vi "OPC UA Client.vi"(11 "?":T9={"VI refs"=[], "Queues"=[], "[Thumbnails]"=[], "Drag Object Idx"=0, "[Objects]"=[], "Active Object"=0, "Drop Offset"={"Left"=0, "Top"=0}, "Process Name"="", "Main Config"={"Notebook"="", "OPC Module Configs"=[], "Feed Module Configs"=[], "Log File Path"=path "", "TT Module Configs"=[], "DAQ Config"={"Tasks"=[]}, "PT Module Configs"=[], "Scale Module Configs"=[], "Pump Module Configs"=[], "U3 Module Configs"=[{"GUID"="", "Drop Coords"={"Horizontal"=0, "Vertical"=0}, "AI Channel Number"=enum."Default", "Process Name"="", "User name"="", "Queue Name"="", "Input Channel Numeric Alarm Settings"=[]}], "Decoration Module Configs"=[], "Flow Module Configs"=[], "TCU Module Configs"=[], "Steps"=[], "Abort"=FALSE, "DO Module Configs"=[], "PR Module Configs"=[], "SC Module Configs"=[], "AM Module Configs"=[], "Cycle Period"=0.0}, "Campaign Filepath"=path "", "Config Changed?"=FALSE} {"Main Config"."PR Module Configs"."Settings"."PID 2 Parameters"."output range"."output low" format="%.2f"; "Main Config"."PR Module Configs"."Settings"."PID 2 Parameters"."output range"."output high" min=0.0 max=100.0 format="%.2f"; "Main Config"."PR Module Configs"."Settings"."PID 2 Parameters"."PID gains"."derivative time (Td, min)" format="%.3f"; "Main Config"."PR Module Configs"."Settings"."PID 2 Parameters"."PID gains"."integral time (Ti, min)" format="%.3f"; "Main Config"."PR Module Configs"."Settings"."PID 2 Parameters"."PID gains"."proportional gain (Kc)" format="%.3f"; "Main Config"."Steps"."Control" items=["Pump %", "Setpoint"]; "Main Config"."TCU Module Configs"."Settings"."Huber Unistat 410 Settings"."Address" min=0 max=99 format="%02.0f"; "Main Config"."TCU Module Configs"."Settings"."Julabo FP-50 Settings"."Pump Power" min=0 max=8 step=1; "Main Config"."TCU Module Configs"."Settings"."Lauda Settings"."Pump Power" min=0 max=8 step=1; "Main Config"."Flow Module Configs"."Settings"."Bronkhorst M14 Settings"."Smoothing Steps" min=1 step=1; "Main Config"."Flow Module Configs"."Settings"."Bronkhorst M13 Settings"."Smoothing Steps" min=1 step=1; "Main Config"."Pump Module Configs"."Settings"."Ismatech 3 Channel Settings"."Channel Number" min=0 max=3; "Main Config"."Pump Module Configs"."Settings"."Ismatech 3 Channel Settings"."Pump Number" min=1; "Main Config"."Pump Module Configs"."Settings"."ASIA Pump C"."channel" min=0 max=1 step=1; "Main Config"."Pump Module Configs"."Settings"."Masterflex"."Pump Number" min=1.0 max=20.0 step=1.0; "Main Config"."Pump Module Configs"."Settings"."Ismatech"."Pump Number" min=1.0 max=20.0 step=1.0; "Main Config"."Feed Module Configs"."Settings"."Bronkhorst M14 Settings"."Smoothing Steps" min=1 step=1; "Main Config"."Feed Module Configs"."Settings"."Ismatech 3 Channel Settings"."Channel Number" min=0 max=3; "Main Config"."Feed Module Configs"."Settings"."Ismatech 3 Channel Settings"."Pump Number" min=1; "Main Config"."Feed Module Configs"."Settings"."output range"."output low" min=0.0 max=100.0 format="%.2f"; "Main Config"."Feed Module Configs"."Settings"."output range"."output high" format="%.2f"; "Main Config"."Feed Module Configs"."Settings"."PID 2 Parameters"."PID gains"."derivative time (Td, min)" format="%.3f"; "Main Config"."Feed Module Configs"."Settings"."PID 2 Parameters"."PID gains"."integral time (Ti, min)" format="%.3f"; "Main Config"."Feed Module Configs"."Settings"."PID 2 Parameters"."PID gains"."proportional gain (Kc)" format="%.3f"; "Main Config"."Feed Module Configs"."Settings"."Bronkhorst M13 Flow Meter"."Smoothing Steps" min=1 step=1; "Main Config"."Feed Module Configs"."Settings"."ASIA Pump C"."channel" min=0 max=1 step=1; "Main Config"."Feed Module Configs"."Settings"."Ismatech"."Pump Number" min=1.0 max=20.0 step=1.0; "Main Config"."Feed Module Configs"."Settings"."Masterflex"."Pump Number" min=1.0 max=20.0 step=1.0}) -> ()   [LabVIEW 2018, in "OPC UA Total Client.lvlib"]
uses:
  OPC UA Total Client.lvlib
  <vilib>/OPCUA/controls/NodeId.ctl
  <vilib>/OPCUA/controls/OPC UA Variable Node Refnum.ctl
  <vilib>/OPCUA/controls/OPC UA Server Refnum.ctl
  Drag and Drop/State Cluster.ctl
  support/Message Queue/Message Cluster.ctl
  Drag and Drop/Thumbnail Cluster.ctl
  Drag and Drop/Object Cluster.ctl
  <vilib>/Utility/miscctls.llb/LVRectTypeDef.ctl
  Drag and Drop/Object Type Enum.ctl
  <vilib>/Utility/miscctls.llb/LVPositionTypeDef.ctl
  Config Module/Controls/Main Config Cluster.ctl
  OPC Module Config.ctl
  Scale Module Folder/Measure Instrument/State Enum.ctl
  <vilib>/Utility/miscctls.llb/LVPoint32TypeDef.ctl
  OPC Settings.ctl
  Variable Data Cluster.ctl
  <vilib>/OPCUA/controls/OPC UA StatusCode.ctl
  <vilib>/OPCUA/controls/Subscription ID.ctl
  <vilib>/OPCUA/controls/OPC UA Client Refnum.ctl
  <vilib>/OPCUA/controls/Subscription Data Change.ctl
  <vilib>/OPCUA/controls/Data Type.ctl
  OPC Tag Data.ctl
  Feed Module/Controls/Feed Module Config Cluster.ctl
  Feed Module/Controls/Feed Module Settings Cluster.ctl
  Ismatec ISM 831C/Controls/Ismatech ISM831C Settings Cluster.ctl
  Masterflex 7550-30/Controls/Settings Cluster.ctl
  Mettler Toledo/Controls/Settings Cluster.ctl
  Bronkhorst M13 Flow Meter/Settings Cluster.ctl
  Measure Instrument/PID 2 Parameters Cluster.ctl
  Measure Instrument/PID Input Enum.ctl
  Measure Instrument/PID 2 Output Enum.ctl
  Tacmina QI/Tacmina QI DAQ Setting.ctl
  KNF Pump/Settings Cluster plus SIMDOS.ctl
  ASIA Pump/Pump Settings.ctl
  VICI M50 Party Mode/Settings Cluster.ctl
  FLOM Pump/Settings Cluster.ctl
  SSI PR Class/SSI PR or LD Settings Cluster.ctl
  Masterflex 75211/Masterflex 75211 DAQ Setting.ctl
  SSI PR Class/SSI P40 Settings Cluster.ctl
  Ismatec 78001/Ismatec 4083.ctl
  Bronkhorst M14 Flow Meter/Settings Cluster.ctl
  TT Module/Controls/TT Module Config Cluster.ctl
  Tag VIs/Numeric Alarm Settings Cluster.ctl
  Acquisition/Hardware Configuration.ctl
  Acquisition/Task Cluster.ctl
  PT Module/Controls/PT Module Config Cluster.ctl
  Scale Module Folder/Feed Module/Controls/Scale Module Config Cluster.ctl
  Scale Module Folder/Feed Module/Controls/Scale Module Settings Cluster.ctl
  Pump Module Folder/Pump Module Config Cluster.ctl
  Pump Module Folder/Pump Module Settings Cluster.ctl
  LabJack Module/Controls/U3 Module Config Cluster.ctl
  Decoration Module/Decoration Module Config Cluster.ctl
  Flow Module Folder/Feed Module/Controls/Flow Module Config Cluster.ctl
  Flow Module Folder/Feed Module/Controls/Flow Module Settings Cluster.ctl
  TCU Module/TCU Module Folder/TCU Module Config Cluster.ctl
  TCU Module/TCU Module Folder/TCU Module Settings Cluster.ctl
  TCU Module/TCU Module Folder/Measure Instrument/Output Devices.ctl
  Huber TCU/Huber Settings.ctl
  Lauda Integral XT-150 TCU/Lauda Settings.ctl
  Julabo Type 1 TCU/Julabo Type 1 TCU Folder/Julabo FP-50 Settings.ctl
  Huber Unistat 410 TCU/Huber Unistat 410 RS485 Settings.ctl
  D-O Module Folder/Not Sure Where this is Used.ctl
  Sequencing/Squence Control.ctl
  D-O Module Folder/D-O Module Config Cluster.ctl
  D-O Module Folder/Valve Clusters.ctl
  D-O Module Folder/D-O Module Settings Cluster.ctl
  D-O Module Folder/D-O Device Settings Cluster.ctl
  VICI Electronic Actuator/VICI Electronic Actuator Settings.ctl
  Pressure Regulator Control Module/Pressure Regulator/Controls/4-20mA Module Config Cluster.ctl
  Pressure Regulator Control Module/Pressure Regulator/Controls/4-20mA Module Settings Cluster.ctl
  Pressure Transmitter/Pressure Transmitter Device Settings.ctl
  Pressure Reg Module/Pressure Regulator Device Settings.ctl
  Sonicator Module Folder/Feed Module/Controls/Sonicator Module Config Cluster.ctl
  Sonicator Module Folder/Feed Module/Controls/Sonicator Module Settings Cluster.ctl
  Sonic Systems P100/Sonic Systems P100 Settings.ctl
  Agitator Module Folder/Feed Module/Controls/Agitator Module Config Cluster.ctl
  Agitator Module Folder/Feed Module/Controls/Agitator Module Settings Cluster.ctl
  <vilib>/OPCUA/controls/Supported Security Policies.ctl
  Main/Main Queue Cluster.ctl
  <vilib>/OPCUA/controls/Read Variant Result.ctl
  <vilib>/OPCUA/controls/Node Class.ctl
  <vilib>/OPCUA/controls/NodeIds.ctl
  <vilib>/OPCUA/client/Multiple Read Variant.vi
  <vilib>/OPCUA/NI OPC UA Server.lvlib
  <vilib>/regexp/Match Regular Expression.xnode
  OPC UA.lvlib
  Tag VIs/Tag FGV Operation Enum.ctl
  Shared Variables/Dynamic Shared Variables.lvlib
  support/Message Queue/Message Queue.lvlib
  <vilib>/OPCUA/NI OPC UA Client.lvlib
  <vilib>/OPCUA/controls/Write Status.ctl
  <vilib>/OPCUA/controls/Write Variant Request.ctl
  <vilib>/OPCUA/server/Write Double.vi
  <vilib>/OPCUA/client/Multiple Write Variant.vi
  support/Message Queue/Enqueue Message (Single).vi
  <vilib>/OPCUA/client/Multiple Write Int32.vi
  TT Module/TT Module.lvlib
  Masterflex 75211/Masterflex 75211.lvlib
  Masterflex 7550-30/Masterflex 7550-30.lvlib
  Ismatec ISM 831C/Ismatec ISM 831C.lvlib
  Tacmina QI/Tacmina QI.lvlib
  KNF Pump/KNF SIMDOS.lvlib
  VICI M50 Party Mode/VICI M6 M50 Party Mode.lvlib
  FLOM Pump/FLOM Pump.lvlib
  ASIA Pump.lvlib
  Mettler Toledo/Mettler Toledo.lvlib
  Bronkhorst M13 Flow Meter/Bronkhorst M13 Flow Meter.lvlib
  SSI PR Class/SSI PR or LD Pump.lvlib
  SSI PR Class/SSI P40 Pump.lvlib
  Feed Module/Feed Module.lvlib
  DAQ/DAQ.lvlib
  PT Module/PT Module.lvlib
  Scale Module Folder/Scale Module.lvlib
  Pump Module Folder/Pump Module.lvlib
  LabJack Module/U3 Module.lvlib
  Flow Module Folder/Flow Module.lvlib
  Huber TCU/Huber Ministat 230 TCU.lvlib
  Lauda Integral XT-150 TCU/Lauda TCU.lvlib
  Julabo Type 1 TCU/Julabo Type 1 TCU Folder/Julabo Type FP-50 TCU.lvlib
  Huber Unistat 410 TCU/Huber Unistat 410 TCU.lvlib
  TCU Module/TCU Module Folder/TCU Module.lvlib
  Sequencing/Sequencing Library.lvlib
  D-O Module Folder/D-O Module.lvlib
  D-O Module Folder/DIO Valve/VICI Electronic Actuator.lvlib
  Pressure Transmitter/Pressure Transmitter Library.lvlib
  Pressure Reg Module/Pressure Regulator Library.lvlib
  Pressure Regulator Control Module/Pressure Regulator/4-20mA Module.lvlib
  Scale Module Folder/Measure Instrument/Scale Module Engine.lvlib
  Config Module/Config Module.lvlib
  Drag and Drop/Drag and Drop.lvlib
  Ismatec 78001/Ismatec 4308.lvlib
  Bronkhorst M14 Flow Meter/Bronkhorst M14 Flow Meter.lvlib
  Sonicator Module Folder/Sonicator Module.lvlib
  Sonic Systems P100/Sonic Systems P100.lvlib
  Agitator Module Folder/Agitator Module.lvlib
panel:
  out "results 2":T1[](array[typedef]) {"status" items=["Good"=0, "Good_SubscriptionTransferred"=2949120, "Good_CompletesAsynchronously"=3014656, "Good_Overload"=3080192, "Good_Clamped"=3145728, "Good_LocalOverride"=9830400, "Good_EntryInserted"=10616832, "Good_EntryReplaced"=10682368, "Good_NoData"=10813440, "Good_MoreData"=10878976, "Good_CommunicationEvent"=10944512, "Good_ShutdownEvent"=11010048, "Good_CallAgain"=11075584, "Good_NonCriticalTimeout"=11141120, "Good_ResultsMayBeIncomplete"=12189696, "Good_DataIgnored"=14221312, "Uncertain"=1073741824, "Uncertain_ReferenceOutOfServer"=1080819712, "Uncertain_NoCommunicationLastUsableValue"=1083113472, "Uncertain_LastUsableValue"=1083179008, "Uncertain_SubstituteValue"=1083244544, "Uncertain_InitialValue"=1083310080, "Uncertain_SensorNotAccurate"=1083375616, "Uncertain_EngineeringUnitsExceeded"=1083441152, "Uncertain_SubNormal"=1083506688, "Uncertain_DataSubNormal"=1084489728, "Uncertain_ReferenceNotDeleted"=1086062592, "Uncertain_NotAllNodesAvailable"=1086324736, "Bad"=2147483648, "Bad_UnexpectedError"=2147549184, "Bad_InternalError"=2147614720, "Bad_OutOfMemory"=2147680256, "Bad_ResourceUnavailable"=2147745792, "Bad_CommunicationError"=2147811328, "Bad_EncodingError"=2147876864, "Bad_DecodingError"=2147942400, "Bad_EncodingLimitsExceeded"=2148007936, "Bad_UnknownResponse"=2148073472, "Bad_Timeout"=2148139008, "Bad_ServiceUnsupported"=2148204544, "Bad_Shutdown"=2148270080, "Bad_ServerNotConnected"=2148335616, "Bad_ServerHalted"=2148401152, "Bad_NothingToDo"=2148466688, "Bad_TooManyOperations"=2148532224, "Bad_DataTypeIdUnknown"=2148597760, "Bad_CertificateInvalid"=2148663296, "Bad_SecurityChecksFailed"=2148728832, "Bad_CertificateTimeInvalid"=2148794368, "Bad_CertificateIssuerTimeInvalid"=2148859904, "Bad_CertificateHostNameInvalid"=2148925440, "Bad_CertificateUriInvalid"=2148990976, "Bad_CertificateUseNotAllowed"=2149056512, "Bad_CertificateIssuerUseNotAllowed"=2149122048, "Bad_CertificateUntrusted"=2149187584, "Bad_CertificateRevocationUnknown"=2149253120, "Bad_CertificateIssuerRevocationUnknown"=2149318656, "Bad_CertificateRevoked"=2149384192, "Bad_CertificateIssuerRevoked"=2149449728, "Bad_UserAccessDenied"=2149515264, "Bad_IdentityTokenInvalid"=2149580800, "Bad_IdentityTokenRejected"=2149646336, "Bad_SecureChannelIdInvalid"=2149711872, "Bad_InvalidTimestamp"=2149777408, "Bad_NonceInvalid"=2149842944, "Bad_SessionIdInvalid"=2149908480, "Bad_SessionClosed"=2149974016, "Bad_SessionNotActivated"=2150039552, "Bad_SubscriptionIdInvalid"=2150105088, "Bad_RequestHeaderInvalid"=2150236160, "Bad_TimestampsToReturnInvalid"=2150301696, "Bad_RequestCancelledByClient"=2150367232, "Bad_NoCommunication"=2150694912, "Bad_WaitingForInitialData"=2150760448, "Bad_NodeIdInvalid"=2150825984, "Bad_NodeIdUnknown"=2150891520, "Bad_AttributeIdInvalid"=2150957056, "Bad_IndexRangeInvalid"=2151022592, "Bad_IndexRangeNoData"=2151088128, "Bad_DataEncodingInvalid"=2151153664, "Bad_DataEncodingUnsupported"=2151219200, "Bad_NotReadable"=2151284736, "Bad_NotWritable"=2151350272, "Bad_OutOfRange"=2151415808, "Bad_NotSupported"=2151481344, "Bad_NotFound"=2151546880, "Bad_ObjectDeleted"=2151612416, "Bad_NotImplemented"=2151677952, "Bad_MonitoringModeInvalid"=2151743488, "Bad_MonitoredItemIdInvalid"=2151809024, "Bad_MonitoredItemFilterInvalid"=2151874560, "Bad_MonitoredItemFilterUnsupported"=2151940096, "Bad_FilterNotAllowed"=2152005632, "Bad_StructureMissing"=2152071168, "Bad_EventFilterInvalid"=2152136704, "Bad_ContentFilterInvalid"=2152202240, "Bad_FilterOperandInvalid"=2152267776, "Bad_ContinuationPointInvalid"=2152333312, "Bad_NoContinuationPoints"=2152398848, "Bad_ReferenceTypeIdInvalid"=2152464384, "Bad_BrowseDirectionInvalid"=2152529920, "Bad_NodeNotInView"=2152595456, "Bad_ServerUriInvalid"=2152660992, "Bad_ServerNameMissing"=2152726528, "Bad_DiscoveryUrlMissing"=2152792064, "Bad_SempahoreFileMissing"=2152857600, "Bad_RequestTypeInvalid"=2152923136, "Bad_SecurityModeRejected"=2152988672, "Bad_SecurityPolicyRejected"=2153054208, "Bad_TooManySessions"=2153119744, "Bad_UserSignatureInvalid"=2153185280, "Bad_ApplicationSignatureInvalid"=2153250816, "Bad_NoValidCertificates"=2153316352, "Bad_RequestCancelledByRequest"=2153381888, "Bad_ParentNodeIdInvalid"=2153447424, "Bad_ReferenceNotAllowed"=2153512960, "Bad_NodeIdRejected"=2153578496, "Bad_NodeIdExists"=2153644032, "Bad_NodeClassInvalid"=2153709568, "Bad_BrowseNameInvalid"=2153775104, "Bad_BrowseNameDuplicated"=2153840640, "Bad_NodeAttributesInvalid"=2153906176, "Bad_TypeDefinitionInvalid"=2153971712, "Bad_SourceNodeIdInvalid"=2154037248, "Bad_TargetNodeIdInvalid"=2154102784, "Bad_DuplicateReferenceNotAllowed"=2154168320, "Bad_InvalidSelfReference"=2154233856, "Bad_ReferenceLocalOnly"=2154299392, "Bad_NoDeleteRights"=2154364928, "Bad_ServerIndexInvalid"=2154430464, "Bad_ViewIdUnknown"=2154496000, "Bad_TooManyMatches"=2154627072, "Bad_QueryTooComplex"=2154692608, "Bad_NoMatch"=2154758144, "Bad_MaxAgeInvalid"=2154823680, "Bad_HistoryOperationInvalid"=2154889216, "Bad_HistoryOperationUnsupported"=2154954752, "Bad_WriteNotSupported"=2155020288, "Bad_TypeMismatch"=2155085824, "Bad_MethodInvalid"=2155151360, "Bad_ArgumentsMissing"=2155216896, "Bad_TooManySubscriptions"=2155282432, "Bad_TooManyPublishRequests"=2155347968, "Bad_NoSubscription"=2155413504, "Bad_SequenceNumberUnknown"=2155479040, "Bad_MessageNotAvailable"=2155544576, "Bad_InsufficientClientProfile"=2155610112, "Bad_TcpServerTooBusy"=2155675648, "Bad_TcpMessageTypeInvalid"=2155741184, "Bad_TcpSecureChannelUnknown"=2155806720, "Bad_TcpMessageTooLarge"=2155872256, "Bad_TcpNotEnoughResources"=2155937792, "Bad_TcpInternalError"=2156003328, "Bad_TcpEndpointUrlInvalid"=2156068864, "Bad_RequestInterrupted"=2156134400, "Bad_RequestTimeout"=2156199936, "Bad_SecureChannelClosed"=2156265472, "Bad_SecureChannelTokenUnknown"=2156331008, "Bad_SequenceNumberInvalid"=2156396544, "Bad_ConfigurationError"=2156462080, "Bad_NotConnected"=2156527616, "Bad_DeviceFailure"=2156593152, "Bad_SensorFailure"=2156658688, "Bad_OutOfService"=2156724224, "Bad_DeadbandFilterInvalid"=2156789760, "Bad_RefreshInProgress"=2157379584, "Bad_ConditionAlreadyDisabled"=2157445120, "Bad_ConditionDisabled"=2157510656, "Bad_EventIdUnknown"=2157576192, "Bad_NoData"=2157641728, "Bad_DataLost"=2157772800, "Bad_DataUnavailable"=2157838336, "Bad_EntryExists"=2157903872, "Bad_NoEntryExists"=2157969408, "Bad_TimestampNotSupported"=2158034944, "Bad_InvalidArgument"=2158690304, "Bad_ConnectionRejected"=2158755840, "Bad_Disconnect"=2158821376, "Bad_ConnectionClosed"=2158886912, "Bad_InvalidState"=2158952448, "Bad_EndOfStream"=2159017984, "Bad_NoDataAvailable"=2159083520, "Bad_WaitingForResponse"=2159149056, "Bad_OperationAbandoned"=2159214592, "Bad_ExpectedStreamToBlock"=2159280128, "Bad_WouldBlock"=2159345664, "Bad_SyntaxError"=2159411200, "Bad_MaxConnectionsReached"=2159476736, "Bad_RequestTooLarge"=2159542272, "Bad_ResponseTooLarge"=2159607808, "Bad_EventNotAcknowledgeable"=2159738880, "Bad_InvalidTimestampArgument"=2159869952, "Bad_ProtocolVersionUnsupported"=2159935488, "Bad_StateNotActive"=2160001024, "Bad_FilterOperatorInvalid"=2160132096, "Bad_FilterOperatorUnsupported"=2160197632, "Bad_FilterOperandCountMismatch"=2160263168, "Bad_FilterElementInvalid"=2160328704, "Bad_FilterLiteralInvalid"=2160394240, "Bad_IdentityChangeNotSupported"=2160459776, "Bad_NotTypeDefinition"=2160590848, "Bad_ViewTimestampInvalid"=2160656384, "Bad_ViewParameterMismatch"=2160721920, "Bad_ViewVersionInvalid"=2160787456, "Bad_ConditionAlreadyEnabled"=2160852992, "Bad_DialogNotActive"=2160918528, "Bad_DialogResponseInvalid"=2160984064, "Bad_ConditionBranchAlreadyAcked"=2161049600, "Bad_ConditionBranchAlreadyConfirmed"=2161115136, "Bad_ConditionAlreadyShelved"=2161180672, "Bad_ConditionNotShelved"=2161246208, "Bad_ShelvingTimeOutOfRange"=2161311744, "Bad_AggregateListMismatch"=2161377280, "Bad_AggregateNotSupported"=2161442816, "Bad_AggregateInvalidInputs"=2161508352, "Bad_BoundNotFound"=2161573888, "Bad_BoundNotSupported"=2161639424, "Bad_AggregateConfigurationRejected"=2161770496, "Bad_TooManyMonitoredItems"=2161836032]}
  out "browse result":T5(array[cluster]) {"node class" items=["Unspecified"=0, "Object"=1, "Variable"=2, "Method"=4, "Object Type"=8, "Variable Type"=16, "Reference Type"=32, "Data Type"=64, "View"=128]}
  out "results":T1[](array[typedef]) {"status" items=["Good"=0, "Good_SubscriptionTransferred"=2949120, "Good_CompletesAsynchronously"=3014656, "Good_Overload"=3080192, "Good_Clamped"=3145728, "Good_LocalOverride"=9830400, "Good_EntryInserted"=10616832, "Good_EntryReplaced"=10682368, "Good_NoData"=10813440, "Good_MoreData"=10878976, "Good_CommunicationEvent"=10944512, "Good_ShutdownEvent"=11010048, "Good_CallAgain"=11075584, "Good_NonCriticalTimeout"=11141120, "Good_ResultsMayBeIncomplete"=12189696, "Good_DataIgnored"=14221312, "Uncertain"=1073741824, "Uncertain_ReferenceOutOfServer"=1080819712, "Uncertain_NoCommunicationLastUsableValue"=1083113472, "Uncertain_LastUsableValue"=1083179008, "Uncertain_SubstituteValue"=1083244544, "Uncertain_InitialValue"=1083310080, "Uncertain_SensorNotAccurate"=1083375616, "Uncertain_EngineeringUnitsExceeded"=1083441152, "Uncertain_SubNormal"=1083506688, "Uncertain_DataSubNormal"=1084489728, "Uncertain_ReferenceNotDeleted"=1086062592, "Uncertain_NotAllNodesAvailable"=1086324736, "Bad"=2147483648, "Bad_UnexpectedError"=2147549184, "Bad_InternalError"=2147614720, "Bad_OutOfMemory"=2147680256, "Bad_ResourceUnavailable"=2147745792, "Bad_CommunicationError"=2147811328, "Bad_EncodingError"=2147876864, "Bad_DecodingError"=2147942400, "Bad_EncodingLimitsExceeded"=2148007936, "Bad_UnknownResponse"=2148073472, "Bad_Timeout"=2148139008, "Bad_ServiceUnsupported"=2148204544, "Bad_Shutdown"=2148270080, "Bad_ServerNotConnected"=2148335616, "Bad_ServerHalted"=2148401152, "Bad_NothingToDo"=2148466688, "Bad_TooManyOperations"=2148532224, "Bad_DataTypeIdUnknown"=2148597760, "Bad_CertificateInvalid"=2148663296, "Bad_SecurityChecksFailed"=2148728832, "Bad_CertificateTimeInvalid"=2148794368, "Bad_CertificateIssuerTimeInvalid"=2148859904, "Bad_CertificateHostNameInvalid"=2148925440, "Bad_CertificateUriInvalid"=2148990976, "Bad_CertificateUseNotAllowed"=2149056512, "Bad_CertificateIssuerUseNotAllowed"=2149122048, "Bad_CertificateUntrusted"=2149187584, "Bad_CertificateRevocationUnknown"=2149253120, "Bad_CertificateIssuerRevocationUnknown"=2149318656, "Bad_CertificateRevoked"=2149384192, "Bad_CertificateIssuerRevoked"=2149449728, "Bad_UserAccessDenied"=2149515264, "Bad_IdentityTokenInvalid"=2149580800, "Bad_IdentityTokenRejected"=2149646336, "Bad_SecureChannelIdInvalid"=2149711872, "Bad_InvalidTimestamp"=2149777408, "Bad_NonceInvalid"=2149842944, "Bad_SessionIdInvalid"=2149908480, "Bad_SessionClosed"=2149974016, "Bad_SessionNotActivated"=2150039552, "Bad_SubscriptionIdInvalid"=2150105088, "Bad_RequestHeaderInvalid"=2150236160, "Bad_TimestampsToReturnInvalid"=2150301696, "Bad_RequestCancelledByClient"=2150367232, "Bad_NoCommunication"=2150694912, "Bad_WaitingForInitialData"=2150760448, "Bad_NodeIdInvalid"=2150825984, "Bad_NodeIdUnknown"=2150891520, "Bad_AttributeIdInvalid"=2150957056, "Bad_IndexRangeInvalid"=2151022592, "Bad_IndexRangeNoData"=2151088128, "Bad_DataEncodingInvalid"=2151153664, "Bad_DataEncodingUnsupported"=2151219200, "Bad_NotReadable"=2151284736, "Bad_NotWritable"=2151350272, "Bad_OutOfRange"=2151415808, "Bad_NotSupported"=2151481344, "Bad_NotFound"=2151546880, "Bad_ObjectDeleted"=2151612416, "Bad_NotImplemented"=2151677952, "Bad_MonitoringModeInvalid"=2151743488, "Bad_MonitoredItemIdInvalid"=2151809024, "Bad_MonitoredItemFilterInvalid"=2151874560, "Bad_MonitoredItemFilterUnsupported"=2151940096, "Bad_FilterNotAllowed"=2152005632, "Bad_StructureMissing"=2152071168, "Bad_EventFilterInvalid"=2152136704, "Bad_ContentFilterInvalid"=2152202240, "Bad_FilterOperandInvalid"=2152267776, "Bad_ContinuationPointInvalid"=2152333312, "Bad_NoContinuationPoints"=2152398848, "Bad_ReferenceTypeIdInvalid"=2152464384, "Bad_BrowseDirectionInvalid"=2152529920, "Bad_NodeNotInView"=2152595456, "Bad_ServerUriInvalid"=2152660992, "Bad_ServerNameMissing"=2152726528, "Bad_DiscoveryUrlMissing"=2152792064, "Bad_SempahoreFileMissing"=2152857600, "Bad_RequestTypeInvalid"=2152923136, "Bad_SecurityModeRejected"=2152988672, "Bad_SecurityPolicyRejected"=2153054208, "Bad_TooManySessions"=2153119744, "Bad_UserSignatureInvalid"=2153185280, "Bad_ApplicationSignatureInvalid"=2153250816, "Bad_NoValidCertificates"=2153316352, "Bad_RequestCancelledByRequest"=2153381888, "Bad_ParentNodeIdInvalid"=2153447424, "Bad_ReferenceNotAllowed"=2153512960, "Bad_NodeIdRejected"=2153578496, "Bad_NodeIdExists"=2153644032, "Bad_NodeClassInvalid"=2153709568, "Bad_BrowseNameInvalid"=2153775104, "Bad_BrowseNameDuplicated"=2153840640, "Bad_NodeAttributesInvalid"=2153906176, "Bad_TypeDefinitionInvalid"=2153971712, "Bad_SourceNodeIdInvalid"=2154037248, "Bad_TargetNodeIdInvalid"=2154102784, "Bad_DuplicateReferenceNotAllowed"=2154168320, "Bad_InvalidSelfReference"=2154233856, "Bad_ReferenceLocalOnly"=2154299392, "Bad_NoDeleteRights"=2154364928, "Bad_ServerIndexInvalid"=2154430464, "Bad_ViewIdUnknown"=2154496000, "Bad_TooManyMatches"=2154627072, "Bad_QueryTooComplex"=2154692608, "Bad_NoMatch"=2154758144, "Bad_MaxAgeInvalid"=2154823680, "Bad_HistoryOperationInvalid"=2154889216, "Bad_HistoryOperationUnsupported"=2154954752, "Bad_WriteNotSupported"=2155020288, "Bad_TypeMismatch"=2155085824, "Bad_MethodInvalid"=2155151360, "Bad_ArgumentsMissing"=2155216896, "Bad_TooManySubscriptions"=2155282432, "Bad_TooManyPublishRequests"=2155347968, "Bad_NoSubscription"=2155413504, "Bad_SequenceNumberUnknown"=2155479040, "Bad_MessageNotAvailable"=2155544576, "Bad_InsufficientClientProfile"=2155610112, "Bad_TcpServerTooBusy"=2155675648, "Bad_TcpMessageTypeInvalid"=2155741184, "Bad_TcpSecureChannelUnknown"=2155806720, "Bad_TcpMessageTooLarge"=2155872256, "Bad_TcpNotEnoughResources"=2155937792, "Bad_TcpInternalError"=2156003328, "Bad_TcpEndpointUrlInvalid"=2156068864, "Bad_RequestInterrupted"=2156134400, "Bad_RequestTimeout"=2156199936, "Bad_SecureChannelClosed"=2156265472, "Bad_SecureChannelTokenUnknown"=2156331008, "Bad_SequenceNumberInvalid"=2156396544, "Bad_ConfigurationError"=2156462080, "Bad_NotConnected"=2156527616, "Bad_DeviceFailure"=2156593152, "Bad_SensorFailure"=2156658688, "Bad_OutOfService"=2156724224, "Bad_DeadbandFilterInvalid"=2156789760, "Bad_RefreshInProgress"=2157379584, "Bad_ConditionAlreadyDisabled"=2157445120, "Bad_ConditionDisabled"=2157510656, "Bad_EventIdUnknown"=2157576192, "Bad_NoData"=2157641728, "Bad_DataLost"=2157772800, "Bad_DataUnavailable"=2157838336, "Bad_EntryExists"=2157903872, "Bad_NoEntryExists"=2157969408, "Bad_TimestampNotSupported"=2158034944, "Bad_InvalidArgument"=2158690304, "Bad_ConnectionRejected"=2158755840, "Bad_Disconnect"=2158821376, "Bad_ConnectionClosed"=2158886912, "Bad_InvalidState"=2158952448, "Bad_EndOfStream"=2159017984, "Bad_NoDataAvailable"=2159083520, "Bad_WaitingForResponse"=2159149056, "Bad_OperationAbandoned"=2159214592, "Bad_ExpectedStreamToBlock"=2159280128, "Bad_WouldBlock"=2159345664, "Bad_SyntaxError"=2159411200, "Bad_MaxConnectionsReached"=2159476736, "Bad_RequestTooLarge"=2159542272, "Bad_ResponseTooLarge"=2159607808, "Bad_EventNotAcknowledgeable"=2159738880, "Bad_InvalidTimestampArgument"=2159869952, "Bad_ProtocolVersionUnsupported"=2159935488, "Bad_StateNotActive"=2160001024, "Bad_FilterOperatorInvalid"=2160132096, "Bad_FilterOperatorUnsupported"=2160197632, "Bad_FilterOperandCountMismatch"=2160263168, "Bad_FilterElementInvalid"=2160328704, "Bad_FilterLiteralInvalid"=2160394240, "Bad_IdentityChangeNotSupported"=2160459776, "Bad_NotTypeDefinition"=2160590848, "Bad_ViewTimestampInvalid"=2160656384, "Bad_ViewParameterMismatch"=2160721920, "Bad_ViewVersionInvalid"=2160787456, "Bad_ConditionAlreadyEnabled"=2160852992, "Bad_DialogNotActive"=2160918528, "Bad_DialogResponseInvalid"=2160984064, "Bad_ConditionBranchAlreadyAcked"=2161049600, "Bad_ConditionBranchAlreadyConfirmed"=2161115136, "Bad_ConditionAlreadyShelved"=2161180672, "Bad_ConditionNotShelved"=2161246208, "Bad_ShelvingTimeOutOfRange"=2161311744, "Bad_AggregateListMismatch"=2161377280, "Bad_AggregateNotSupported"=2161442816, "Bad_AggregateInvalidInputs"=2161508352, "Bad_BoundNotFound"=2161573888, "Bad_BoundNotSupported"=2161639424, "Bad_AggregateConfigurationRejected"=2161770496, "Bad_TooManyMonitoredItems"=2161836032]}
  in  "OPC UA server name":string=" 10.131.0.142:49580"
  in  "security policy 2":T6={"message mode"=enum."Sign", "security"=enum."Basic256"}
  in  "security policy":T6={"message mode"=enum."Sign", "security"=enum."Basic256"}
  out "Waveform Chart":i32(graph)
  out "data change":T7[](array[typedef]) {"data type" items=["Boolean"=1, "SByte"=2, "Byte"=3, "Int16"=4, "UInt16"=5, "Int32"=6, "UInt32"=7, "Int64"=8, "UInt64"=9, "Float"=10, "Double"=11, "String"=12, "DateTime"=13, "ByteString"=15, "Array of Boolean"=101, "Array of SByte"=102, "Array of Byte"=103, "Array of Int16"=104, "Array of UInt16"=105, "Array of Int32"=106, "Array of UInt32"=107, "Array of Int64"=108, "Array of UInt64"=109, "Array of Float"=110, "Array of Double"=111, "Array of String"=112, "Array of DateTime"=113, "Array of ByteString"=115, "Matrix of Boolean"=201, "Matrix of SByte"=202, "Matrix of Byte"=203, "Matrix of Int16"=204, "Matrix of UInt16"=205, "Matrix of Int32"=206, "Matrix of UInt32"=207, "Matrix of Int64"=208, "Matrix of UInt64"=209, "Matrix of Float"=210, "Matrix of Double"=211, "Matrix of String "=212, "Matrix of DateTime"=213, "Matrix of ByteString"=215]; "status code" items=["Good"=0, "Good_SubscriptionTransferred"=2949120, "Good_CompletesAsynchronously"=3014656, "Good_Overload"=3080192, "Good_Clamped"=3145728, "Good_LocalOverride"=9830400, "Good_EntryInserted"=10616832, "Good_EntryReplaced"=10682368, "Good_NoData"=10813440, "Good_MoreData"=10878976, "Good_CommunicationEvent"=10944512, "Good_ShutdownEvent"=11010048, "Good_CallAgain"=11075584, "Good_NonCriticalTimeout"=11141120, "Good_ResultsMayBeIncomplete"=12189696, "Good_DataIgnored"=14221312, "Uncertain"=1073741824, "Uncertain_ReferenceOutOfServer"=1080819712, "Uncertain_NoCommunicationLastUsableValue"=1083113472, "Uncertain_LastUsableValue"=1083179008, "Uncertain_SubstituteValue"=1083244544, "Uncertain_InitialValue"=1083310080, "Uncertain_SensorNotAccurate"=1083375616, "Uncertain_EngineeringUnitsExceeded"=1083441152, "Uncertain_SubNormal"=1083506688, "Uncertain_DataSubNormal"=1084489728, "Uncertain_ReferenceNotDeleted"=1086062592, "Uncertain_NotAllNodesAvailable"=1086324736, "Bad"=2147483648, "Bad_UnexpectedError"=2147549184, "Bad_InternalError"=2147614720, "Bad_OutOfMemory"=2147680256, "Bad_ResourceUnavailable"=2147745792, "Bad_CommunicationError"=2147811328, "Bad_EncodingError"=2147876864, "Bad_DecodingError"=2147942400, "Bad_EncodingLimitsExceeded"=2148007936, "Bad_UnknownResponse"=2148073472, "Bad_Timeout"=2148139008, "Bad_ServiceUnsupported"=2148204544, "Bad_Shutdown"=2148270080, "Bad_ServerNotConnected"=2148335616, "Bad_ServerHalted"=2148401152, "Bad_NothingToDo"=2148466688, "Bad_TooManyOperations"=2148532224, "Bad_DataTypeIdUnknown"=2148597760, "Bad_CertificateInvalid"=2148663296, "Bad_SecurityChecksFailed"=2148728832, "Bad_CertificateTimeInvalid"=2148794368, "Bad_CertificateIssuerTimeInvalid"=2148859904, "Bad_CertificateHostNameInvalid"=2148925440, "Bad_CertificateUriInvalid"=2148990976, "Bad_CertificateUseNotAllowed"=2149056512, "Bad_CertificateIssuerUseNotAllowed"=2149122048, "Bad_CertificateUntrusted"=2149187584, "Bad_CertificateRevocationUnknown"=2149253120, "Bad_CertificateIssuerRevocationUnknown"=2149318656, "Bad_CertificateRevoked"=2149384192, "Bad_CertificateIssuerRevoked"=2149449728, "Bad_UserAccessDenied"=2149515264, "Bad_IdentityTokenInvalid"=2149580800, "Bad_IdentityTokenRejected"=2149646336, "Bad_SecureChannelIdInvalid"=2149711872, "Bad_InvalidTimestamp"=2149777408, "Bad_NonceInvalid"=2149842944, "Bad_SessionIdInvalid"=2149908480, "Bad_SessionClosed"=2149974016, "Bad_SessionNotActivated"=2150039552, "Bad_SubscriptionIdInvalid"=2150105088, "Bad_RequestHeaderInvalid"=2150236160, "Bad_TimestampsToReturnInvalid"=2150301696, "Bad_RequestCancelledByClient"=2150367232, "Bad_NoCommunication"=2150694912, "Bad_WaitingForInitialData"=2150760448, "Bad_NodeIdInvalid"=2150825984, "Bad_NodeIdUnknown"=2150891520, "Bad_AttributeIdInvalid"=2150957056, "Bad_IndexRangeInvalid"=2151022592, "Bad_IndexRangeNoData"=2151088128, "Bad_DataEncodingInvalid"=2151153664, "Bad_DataEncodingUnsupported"=2151219200, "Bad_NotReadable"=2151284736, "Bad_NotWritable"=2151350272, "Bad_OutOfRange"=2151415808, "Bad_NotSupported"=2151481344, "Bad_NotFound"=2151546880, "Bad_ObjectDeleted"=2151612416, "Bad_NotImplemented"=2151677952, "Bad_MonitoringModeInvalid"=2151743488, "Bad_MonitoredItemIdInvalid"=2151809024, "Bad_MonitoredItemFilterInvalid"=2151874560, "Bad_MonitoredItemFilterUnsupported"=2151940096, "Bad_FilterNotAllowed"=2152005632, "Bad_StructureMissing"=2152071168, "Bad_EventFilterInvalid"=2152136704, "Bad_ContentFilterInvalid"=2152202240, "Bad_FilterOperandInvalid"=2152267776, "Bad_ContinuationPointInvalid"=2152333312, "Bad_NoContinuationPoints"=2152398848, "Bad_ReferenceTypeIdInvalid"=2152464384, "Bad_BrowseDirectionInvalid"=2152529920, "Bad_NodeNotInView"=2152595456, "Bad_ServerUriInvalid"=2152660992, "Bad_ServerNameMissing"=2152726528, "Bad_DiscoveryUrlMissing"=2152792064, "Bad_SempahoreFileMissing"=2152857600, "Bad_RequestTypeInvalid"=2152923136, "Bad_SecurityModeRejected"=2152988672, "Bad_SecurityPolicyRejected"=2153054208, "Bad_TooManySessions"=2153119744, "Bad_UserSignatureInvalid"=2153185280, "Bad_ApplicationSignatureInvalid"=2153250816, "Bad_NoValidCertificates"=2153316352, "Bad_RequestCancelledByRequest"=2153381888, "Bad_ParentNodeIdInvalid"=2153447424, "Bad_ReferenceNotAllowed"=2153512960, "Bad_NodeIdRejected"=2153578496, "Bad_NodeIdExists"=2153644032, "Bad_NodeClassInvalid"=2153709568, "Bad_BrowseNameInvalid"=2153775104, "Bad_BrowseNameDuplicated"=2153840640, "Bad_NodeAttributesInvalid"=2153906176, "Bad_TypeDefinitionInvalid"=2153971712, "Bad_SourceNodeIdInvalid"=2154037248, "Bad_TargetNodeIdInvalid"=2154102784, "Bad_DuplicateReferenceNotAllowed"=2154168320, "Bad_InvalidSelfReference"=2154233856, "Bad_ReferenceLocalOnly"=2154299392, "Bad_NoDeleteRights"=2154364928, "Bad_ServerIndexInvalid"=2154430464, "Bad_ViewIdUnknown"=2154496000, "Bad_TooManyMatches"=2154627072, "Bad_QueryTooComplex"=2154692608, "Bad_NoMatch"=2154758144, "Bad_MaxAgeInvalid"=2154823680, "Bad_HistoryOperationInvalid"=2154889216, "Bad_HistoryOperationUnsupported"=2154954752, "Bad_WriteNotSupported"=2155020288, "Bad_TypeMismatch"=2155085824, "Bad_MethodInvalid"=2155151360, "Bad_ArgumentsMissing"=2155216896, "Bad_TooManySubscriptions"=2155282432, "Bad_TooManyPublishRequests"=2155347968, "Bad_NoSubscription"=2155413504, "Bad_SequenceNumberUnknown"=2155479040, "Bad_MessageNotAvailable"=2155544576, "Bad_InsufficientClientProfile"=2155610112, "Bad_TcpServerTooBusy"=2155675648, "Bad_TcpMessageTypeInvalid"=2155741184, "Bad_TcpSecureChannelUnknown"=2155806720, "Bad_TcpMessageTooLarge"=2155872256, "Bad_TcpNotEnoughResources"=2155937792, "Bad_TcpInternalError"=2156003328, "Bad_TcpEndpointUrlInvalid"=2156068864, "Bad_RequestInterrupted"=2156134400, "Bad_RequestTimeout"=2156199936, "Bad_SecureChannelClosed"=2156265472, "Bad_SecureChannelTokenUnknown"=2156331008, "Bad_SequenceNumberInvalid"=2156396544, "Bad_ConfigurationError"=2156462080, "Bad_NotConnected"=2156527616, "Bad_DeviceFailure"=2156593152, "Bad_SensorFailure"=2156658688, "Bad_OutOfService"=2156724224, "Bad_DeadbandFilterInvalid"=2156789760, "Bad_RefreshInProgress"=2157379584, "Bad_ConditionAlreadyDisabled"=2157445120, "Bad_ConditionDisabled"=2157510656, "Bad_EventIdUnknown"=2157576192, "Bad_NoData"=2157641728, "Bad_DataLost"=2157772800, "Bad_DataUnavailable"=2157838336, "Bad_EntryExists"=2157903872, "Bad_NoEntryExists"=2157969408, "Bad_TimestampNotSupported"=2158034944, "Bad_InvalidArgument"=2158690304, "Bad_ConnectionRejected"=2158755840, "Bad_Disconnect"=2158821376, "Bad_ConnectionClosed"=2158886912, "Bad_InvalidState"=2158952448, "Bad_EndOfStream"=2159017984, "Bad_NoDataAvailable"=2159083520, "Bad_WaitingForResponse"=2159149056, "Bad_OperationAbandoned"=2159214592, "Bad_ExpectedStreamToBlock"=2159280128, "Bad_WouldBlock"=2159345664, "Bad_SyntaxError"=2159411200, "Bad_MaxConnectionsReached"=2159476736, "Bad_RequestTooLarge"=2159542272, "Bad_ResponseTooLarge"=2159607808, "Bad_EventNotAcknowledgeable"=2159738880, "Bad_InvalidTimestampArgument"=2159869952, "Bad_ProtocolVersionUnsupported"=2159935488, "Bad_StateNotActive"=2160001024, "Bad_FilterOperatorInvalid"=2160132096, "Bad_FilterOperatorUnsupported"=2160197632, "Bad_FilterOperandCountMismatch"=2160263168, "Bad_FilterElementInvalid"=2160328704, "Bad_FilterLiteralInvalid"=2160394240, "Bad_IdentityChangeNotSupported"=2160459776, "Bad_NotTypeDefinition"=2160590848, "Bad_ViewTimestampInvalid"=2160656384, "Bad_ViewParameterMismatch"=2160721920, "Bad_ViewVersionInvalid"=2160787456, "Bad_ConditionAlreadyEnabled"=2160852992, "Bad_DialogNotActive"=2160918528, "Bad_DialogResponseInvalid"=2160984064, "Bad_ConditionBranchAlreadyAcked"=2161049600, "Bad_ConditionBranchAlreadyConfirmed"=2161115136, "Bad_ConditionAlreadyShelved"=2161180672, "Bad_ConditionNotShelved"=2161246208, "Bad_ShelvingTimeOutOfRange"=2161311744, "Bad_AggregateListMismatch"=2161377280, "Bad_AggregateNotSupported"=2161442816, "Bad_AggregateInvalidInputs"=2161508352, "Bad_BoundNotFound"=2161573888, "Bad_BoundNotSupported"=2161639424, "Bad_AggregateConfigurationRejected"=2161770496, "Bad_TooManyMonitoredItems"=2161836032]}
  in  "stop":bool
  in  "Device.Node.Set Point":i32=1000
  in  "server endpoint URL 2":string="opc.tcp://localhost:49580"
  in  "Main Queue Cluster":T79
  in  "supported security policies (None)":T80={"None"=TRUE, "Sign with Basic128Rsa15"=TRUE, "Sign and Encrypt with Basic128Rsa15"=TRUE, "Sign with Basic256"=TRUE, "Sign and Encrypt with Basic256"=TRUE}
  out "Tag Values":dbl[](array[numeric])
  out "Tag Names":string[](array[string])
  out "Array":T82(array[cluster])
  out "OPC UA server refnum out":T83
  out "Array 2":T3[](array[typedef]) items=["Good"=0, "Good_SubscriptionTransferred"=2949120, "Good_CompletesAsynchronously"=3014656, "Good_Overload"=3080192, "Good_Clamped"=3145728, "Good_LocalOverride"=9830400, "Good_EntryInserted"=10616832, "Good_EntryReplaced"=10682368, "Good_NoData"=10813440, "Good_MoreData"=10878976, "Good_CommunicationEvent"=10944512, "Good_ShutdownEvent"=11010048, "Good_CallAgain"=11075584, "Good_NonCriticalTimeout"=11141120, "Good_ResultsMayBeIncomplete"=12189696, "Good_DataIgnored"=14221312, "Uncertain"=1073741824, "Uncertain_ReferenceOutOfServer"=1080819712, "Uncertain_NoCommunicationLastUsableValue"=1083113472, "Uncertain_LastUsableValue"=1083179008, "Uncertain_SubstituteValue"=1083244544, "Uncertain_InitialValue"=1083310080, "Uncertain_SensorNotAccurate"=1083375616, "Uncertain_EngineeringUnitsExceeded"=1083441152, "Uncertain_SubNormal"=1083506688, "Uncertain_DataSubNormal"=1084489728, "Uncertain_ReferenceNotDeleted"=1086062592, "Uncertain_NotAllNodesAvailable"=1086324736, "Bad"=2147483648, "Bad_UnexpectedError"=2147549184, "Bad_InternalError"=2147614720, "Bad_OutOfMemory"=2147680256, "Bad_ResourceUnavailable"=2147745792, "Bad_CommunicationError"=2147811328, "Bad_EncodingError"=2147876864, "Bad_DecodingError"=2147942400, "Bad_EncodingLimitsExceeded"=2148007936, "Bad_UnknownResponse"=2148073472, "Bad_Timeout"=2148139008, "Bad_ServiceUnsupported"=2148204544, "Bad_Shutdown"=2148270080, "Bad_ServerNotConnected"=2148335616, "Bad_ServerHalted"=2148401152, "Bad_NothingToDo"=2148466688, "Bad_TooManyOperations"=2148532224, "Bad_DataTypeIdUnknown"=2148597760, "Bad_CertificateInvalid"=2148663296, "Bad_SecurityChecksFailed"=2148728832, "Bad_CertificateTimeInvalid"=2148794368, "Bad_CertificateIssuerTimeInvalid"=2148859904, "Bad_CertificateHostNameInvalid"=2148925440, "Bad_CertificateUriInvalid"=2148990976, "Bad_CertificateUseNotAllowed"=2149056512, "Bad_CertificateIssuerUseNotAllowed"=2149122048, "Bad_CertificateUntrusted"=2149187584, "Bad_CertificateRevocationUnknown"=2149253120, "Bad_CertificateIssuerRevocationUnknown"=2149318656, "Bad_CertificateRevoked"=2149384192, "Bad_CertificateIssuerRevoked"=2149449728, "Bad_UserAccessDenied"=2149515264, "Bad_IdentityTokenInvalid"=2149580800, "Bad_IdentityTokenRejected"=2149646336, "Bad_SecureChannelIdInvalid"=2149711872, "Bad_InvalidTimestamp"=2149777408, "Bad_NonceInvalid"=2149842944, "Bad_SessionIdInvalid"=2149908480, "Bad_SessionClosed"=2149974016, "Bad_SessionNotActivated"=2150039552, "Bad_SubscriptionIdInvalid"=2150105088, "Bad_RequestHeaderInvalid"=2150236160, "Bad_TimestampsToReturnInvalid"=2150301696, "Bad_RequestCancelledByClient"=2150367232, "Bad_NoCommunication"=2150694912, "Bad_WaitingForInitialData"=2150760448, "Bad_NodeIdInvalid"=2150825984, "Bad_NodeIdUnknown"=2150891520, "Bad_AttributeIdInvalid"=2150957056, "Bad_IndexRangeInvalid"=2151022592, "Bad_IndexRangeNoData"=2151088128, "Bad_DataEncodingInvalid"=2151153664, "Bad_DataEncodingUnsupported"=2151219200, "Bad_NotReadable"=2151284736, "Bad_NotWritable"=2151350272, "Bad_OutOfRange"=2151415808, "Bad_NotSupported"=2151481344, "Bad_NotFound"=2151546880, "Bad_ObjectDeleted"=2151612416, "Bad_NotImplemented"=2151677952, "Bad_MonitoringModeInvalid"=2151743488, "Bad_MonitoredItemIdInvalid"=2151809024, "Bad_MonitoredItemFilterInvalid"=2151874560, "Bad_MonitoredItemFilterUnsupported"=2151940096, "Bad_FilterNotAllowed"=2152005632, "Bad_StructureMissing"=2152071168, "Bad_EventFilterInvalid"=2152136704, "Bad_ContentFilterInvalid"=2152202240, "Bad_FilterOperandInvalid"=2152267776, "Bad_ContinuationPointInvalid"=2152333312, "Bad_NoContinuationPoints"=2152398848, "Bad_ReferenceTypeIdInvalid"=2152464384, "Bad_BrowseDirectionInvalid"=2152529920, "Bad_NodeNotInView"=2152595456, "Bad_ServerUriInvalid"=2152660992, "Bad_ServerNameMissing"=2152726528, "Bad_DiscoveryUrlMissing"=2152792064, "Bad_SempahoreFileMissing"=2152857600, "Bad_RequestTypeInvalid"=2152923136, "Bad_SecurityModeRejected"=2152988672, "Bad_SecurityPolicyRejected"=2153054208, "Bad_TooManySessions"=2153119744, "Bad_UserSignatureInvalid"=2153185280, "Bad_ApplicationSignatureInvalid"=2153250816, "Bad_NoValidCertificates"=2153316352, "Bad_RequestCancelledByRequest"=2153381888, "Bad_ParentNodeIdInvalid"=2153447424, "Bad_ReferenceNotAllowed"=2153512960, "Bad_NodeIdRejected"=2153578496, "Bad_NodeIdExists"=2153644032, "Bad_NodeClassInvalid"=2153709568, "Bad_BrowseNameInvalid"=2153775104, "Bad_BrowseNameDuplicated"=2153840640, "Bad_NodeAttributesInvalid"=2153906176, "Bad_TypeDefinitionInvalid"=2153971712, "Bad_SourceNodeIdInvalid"=2154037248, "Bad_TargetNodeIdInvalid"=2154102784, "Bad_DuplicateReferenceNotAllowed"=2154168320, "Bad_InvalidSelfReference"=2154233856, "Bad_ReferenceLocalOnly"=2154299392, "Bad_NoDeleteRights"=2154364928, "Bad_ServerIndexInvalid"=2154430464, "Bad_ViewIdUnknown"=2154496000, "Bad_TooManyMatches"=2154627072, "Bad_QueryTooComplex"=2154692608, "Bad_NoMatch"=2154758144, "Bad_MaxAgeInvalid"=2154823680, "Bad_HistoryOperationInvalid"=2154889216, "Bad_HistoryOperationUnsupported"=2154954752, "Bad_WriteNotSupported"=2155020288, "Bad_TypeMismatch"=2155085824, "Bad_MethodInvalid"=2155151360, "Bad_ArgumentsMissing"=2155216896, "Bad_TooManySubscriptions"=2155282432, "Bad_TooManyPublishRequests"=2155347968, "Bad_NoSubscription"=2155413504, "Bad_SequenceNumberUnknown"=2155479040, "Bad_MessageNotAvailable"=2155544576, "Bad_InsufficientClientProfile"=2155610112, "Bad_TcpServerTooBusy"=2155675648, "Bad_TcpMessageTypeInvalid"=2155741184, "Bad_TcpSecureChannelUnknown"=2155806720, "Bad_TcpMessageTooLarge"=2155872256, "Bad_TcpNotEnoughResources"=2155937792, "Bad_TcpInternalError"=2156003328, "Bad_TcpEndpointUrlInvalid"=2156068864, "Bad_RequestInterrupted"=2156134400, "Bad_RequestTimeout"=2156199936, "Bad_SecureChannelClosed"=2156265472, "Bad_SecureChannelTokenUnknown"=2156331008, "Bad_SequenceNumberInvalid"=2156396544, "Bad_ConfigurationError"=2156462080, "Bad_NotConnected"=2156527616, "Bad_DeviceFailure"=2156593152, "Bad_SensorFailure"=2156658688, "Bad_OutOfService"=2156724224, "Bad_DeadbandFilterInvalid"=2156789760, "Bad_RefreshInProgress"=2157379584, "Bad_ConditionAlreadyDisabled"=2157445120, "Bad_ConditionDisabled"=2157510656, "Bad_EventIdUnknown"=2157576192, "Bad_NoData"=2157641728, "Bad_DataLost"=2157772800, "Bad_DataUnavailable"=2157838336, "Bad_EntryExists"=2157903872, "Bad_NoEntryExists"=2157969408, "Bad_TimestampNotSupported"=2158034944, "Bad_InvalidArgument"=2158690304, "Bad_ConnectionRejected"=2158755840, "Bad_Disconnect"=2158821376, "Bad_ConnectionClosed"=2158886912, "Bad_InvalidState"=2158952448, "Bad_EndOfStream"=2159017984, "Bad_NoDataAvailable"=2159083520, "Bad_WaitingForResponse"=2159149056, "Bad_OperationAbandoned"=2159214592, "Bad_ExpectedStreamToBlock"=2159280128, "Bad_WouldBlock"=2159345664, "Bad_SyntaxError"=2159411200, "Bad_MaxConnectionsReached"=2159476736, "Bad_RequestTooLarge"=2159542272, "Bad_ResponseTooLarge"=2159607808, "Bad_EventNotAcknowledgeable"=2159738880, "Bad_InvalidTimestampArgument"=2159869952, "Bad_ProtocolVersionUnsupported"=2159935488, "Bad_StateNotActive"=2160001024, "Bad_FilterOperatorInvalid"=2160132096, "Bad_FilterOperatorUnsupported"=2160197632, "Bad_FilterOperandCountMismatch"=2160263168, "Bad_FilterElementInvalid"=2160328704, "Bad_FilterLiteralInvalid"=2160394240, "Bad_IdentityChangeNotSupported"=2160459776, "Bad_NotTypeDefinition"=2160590848, "Bad_ViewTimestampInvalid"=2160656384, "Bad_ViewParameterMismatch"=2160721920, "Bad_ViewVersionInvalid"=2160787456, "Bad_ConditionAlreadyEnabled"=2160852992, "Bad_DialogNotActive"=2160918528, "Bad_DialogResponseInvalid"=2160984064, "Bad_ConditionBranchAlreadyAcked"=2161049600, "Bad_ConditionBranchAlreadyConfirmed"=2161115136, "Bad_ConditionAlreadyShelved"=2161180672, "Bad_ConditionNotShelved"=2161246208, "Bad_ShelvingTimeOutOfRange"=2161311744, "Bad_AggregateListMismatch"=2161377280, "Bad_AggregateNotSupported"=2161442816, "Bad_AggregateInvalidInputs"=2161508352, "Bad_BoundNotFound"=2161573888, "Bad_BoundNotSupported"=2161639424, "Bad_AggregateConfigurationRejected"=2161770496, "Bad_TooManyMonitoredItems"=2161836032]
  out "server endpoint URL":string
  in  "?":T9 {"Main Config"."PR Module Configs"."Settings"."PID 2 Parameters"."output range"."output low" format="%.2f"; "Main Config"."PR Module Configs"."Settings"."PID 2 Parameters"."output range"."output high" min=0.0 max=100.0 format="%.2f"; "Main Config"."PR Module Configs"."Settings"."PID 2 Parameters"."PID gains"."derivative time (Td, min)" format="%.3f"; "Main Config"."PR Module Configs"."Settings"."PID 2 Parameters"."PID gains"."integral time (Ti, min)" format="%.3f"; "Main Config"."PR Module Configs"."Settings"."PID 2 Parameters"."PID gains"."proportional gain (Kc)" format="%.3f"; "Main Config"."Steps"."Control" items=["Pump %", "Setpoint"]; "Main Config"."TCU Module Configs"."Settings"."Huber Unistat 410 Settings"."Address" min=0 max=99 format="%02.0f"; "Main Config"."TCU Module Configs"."Settings"."Julabo FP-50 Settings"."Pump Power" min=0 max=8 step=1; "Main Config"."TCU Module Configs"."Settings"."Lauda Settings"."Pump Power" min=0 max=8 step=1; "Main Config"."Flow Module Configs"."Settings"."Bronkhorst M14 Settings"."Smoothing Steps" min=1 step=1; "Main Config"."Flow Module Configs"."Settings"."Bronkhorst M13 Settings"."Smoothing Steps" min=1 step=1; "Main Config"."Pump Module Configs"."Settings"."Ismatech 3 Channel Settings"."Channel Number" min=0 max=3; "Main Config"."Pump Module Configs"."Settings"."Ismatech 3 Channel Settings"."Pump Number" min=1; "Main Config"."Pump Module Configs"."Settings"."ASIA Pump C"."channel" min=0 max=1 step=1; "Main Config"."Pump Module Configs"."Settings"."Masterflex"."Pump Number" min=1.0 max=20.0 step=1.0; "Main Config"."Pump Module Configs"."Settings"."Ismatech"."Pump Number" min=1.0 max=20.0 step=1.0; "Main Config"."Feed Module Configs"."Settings"."Bronkhorst M14 Settings"."Smoothing Steps" min=1 step=1; "Main Config"."Feed Module Configs"."Settings"."Ismatech 3 Channel Settings"."Channel Number" min=0 max=3; "Main Config"."Feed Module Configs"."Settings"."Ismatech 3 Channel Settings"."Pump Number" min=1; "Main Config"."Feed Module Configs"."Settings"."output range"."output low" min=0.0 max=100.0 format="%.2f"; "Main Config"."Feed Module Configs"."Settings"."output range"."output high" format="%.2f"; "Main Config"."Feed Module Configs"."Settings"."PID 2 Parameters"."PID gains"."derivative time (Td, min)" format="%.3f"; "Main Config"."Feed Module Configs"."Settings"."PID 2 Parameters"."PID gains"."integral time (Ti, min)" format="%.3f"; "Main Config"."Feed Module Configs"."Settings"."PID 2 Parameters"."PID gains"."proportional gain (Kc)" format="%.3f"; "Main Config"."Feed Module Configs"."Settings"."Bronkhorst M13 Flow Meter"."Smoothing Steps" min=1 step=1; "Main Config"."Feed Module Configs"."Settings"."ASIA Pump C"."channel" min=0 max=1 step=1; "Main Config"."Feed Module Configs"."Settings"."Ismatech"."Pump Number" min=1.0 max=20.0 step=1.0; "Main Config"."Feed Module Configs"."Settings"."Masterflex"."Pump Number" min=1.0 max=20.0 step=1.0}
  out "Array 4":T82(array[cluster])
  out "OPC UA server refnum out 3":T83
  out "Array 3":T82(array[cluster])
  # "Agitator Settings"
  # "Sonicator Settings"
  # "Instrument Settings"
  # "Instrument Settings"
  # "Output Instruments"
  # "Flow Meter Settings"
  # "Output Instruments"
  # "Scale Settings"
  # "Output Instruments"
  # "Input Instruments"
  # "Agitator Settings"
  # "Sonicator Settings"
  # "Instrument Settings"
  # "Instrument Settings"
  # "Output Instruments"
  # "Flow Meter Settings"
  # "Output Instruments"
  # "Scale Settings"
  # "Output Instruments"
  # "Input Instruments"
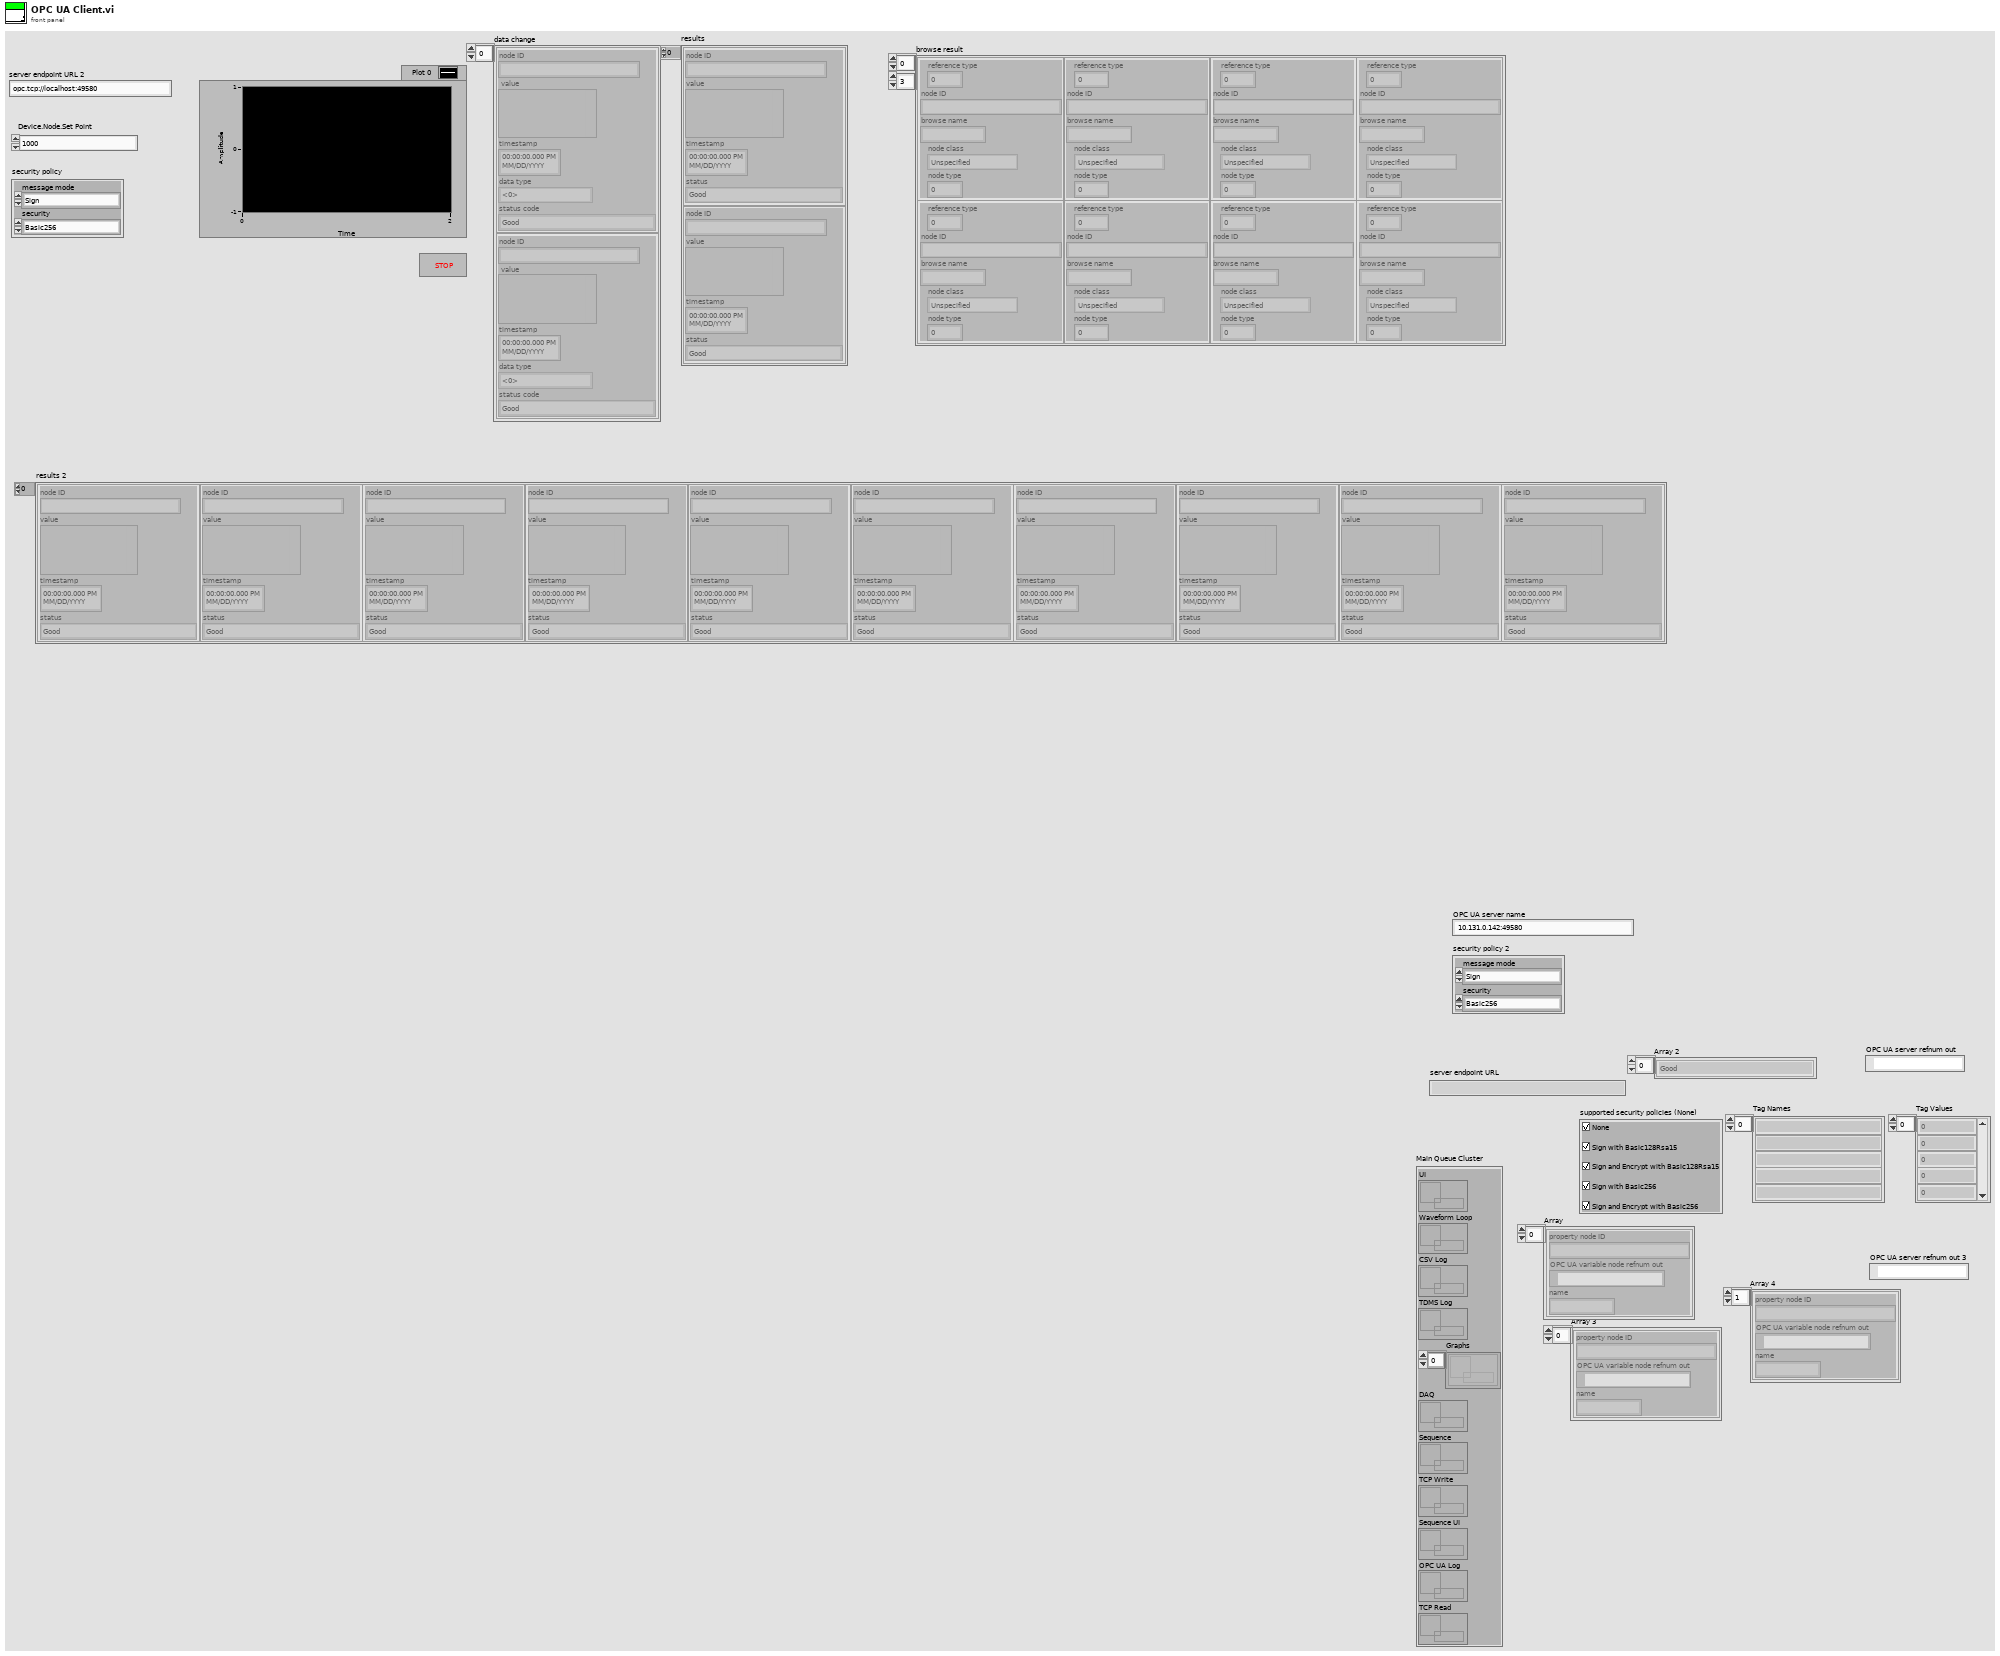
[diagram p1: front panel]
types:
  T1 = typedef "Read Variant Result.ctl" = cluster{"node ID":T2, "value ":variant, "timestamp":timestamp, "status":T3}
  T2 = typedef "NodeId.ctl" = string
  T3 = typedef "OPC UA StatusCode.ctl" = u32
  T4 = typedef "Node Class.ctl" = u32
  T5 = cluster{"reference type":u32, "node ID":T2, "browse name":string, "node class":T4, "node type":u32}[][]
  T6 = cluster{"message mode":enum16{"None", "Sign", "Sign and Encrypt"}, "security":enum16{"Basic256", "Basic128Rsa15"}}
  T7 = typedef "Subscription Data Change.ctl" = cluster{"node ID":T2, " value":variant, "timestamp":timestamp, "data type":T8, "status code":T3}
  T8 = typedef "Data Type.ctl" = u16
  T9 = typedef "Drag and Drop.lvlib/State Cluster.ctl" = cluster{"VI refs":refnum<vi>[], "Queues":refnum<queue>[], "[Thumbnails]":T10[], "Drag Object Idx":i32, "[Objects]":T11[], "Active Object":i32, "Drop Offset":T14, "Process Name":string, "Main Config":T15, "Campaign Filepath":path, "Config Changed?":bool}
  T10 = typedef "Thumbnail Cluster.ctl" = cluster{"Path":path, "Rectangle":cluster{"left":i16, "top":i16, "right":i16, "bottom":i16}}
  T11 = typedef "Object Cluster.ctl" = cluster{"BMP Path":path, "Anchor Position":cluster{"X":i32, "Y":i32}, "Hot Spot":T12, "Type":T13, "Parameters":variant}
  T12 = typedef "LVRectTypeDef.ctl" = cluster{"Left":i16, "Top":i16, "Right":i16, "Bottom":i16}
  T13 = typedef "Object Type Enum.ctl" = enum16{"Icon", "Line", "Text", "Feed Module"}
  T14 = typedef "LVPositionTypeDef.ctl" = cluster{"Left":i32, "Top":i32}
  T15 = typedef "Config Module.lvlib/Main Config Cluster.ctl" = cluster{"Notebook":string, "OPC Module Configs":T16[], "Feed Module Configs":T24[], "Log File Path":path, "TT Module Configs":T43[], "DAQ Config":T45, "PT Module Configs":T47[], "Scale Module Configs":T48[], "Pump Module Configs":T50[], "U3 Module Configs":T52[], "Decoration Module Configs":T53[], "Flow Module Configs":T54[], "TCU Module Configs":T56[], "Steps":T63, "Abort":bool, "DO Module Configs":T65[], "PR Module Configs":T70[], "SC Module Configs":T74[], "AM Module Configs":T77[], "Cycle Period":dbl}
  T16 = typedef "OPC UA.lvlib/OPC Module Config.ctl" = cluster{"State":T17, "GUID":string, "Process Name":string, "User name":string, "Drop Coords":T18, "Configuration":T19, "First Iteration":bool, "Data":cluster{"Object Name":string, "Variable Array":T20[]}[], "Load Count":i32, "Log Started":bool, "subscription ID out":T21, "OPC UA client refnum out":T22, "Event Registration Refnum":refnum<event-registration>, "Start Time":timestamp, "Current Time":timestamp, "Tag Data":T23[]}
  T17 = typedef "Scale Module.lvlib/Scale Module Engine.lvlib/State Enum.ctl" = enum16{"Measuring", "Idle"}
  T18 = typedef "LVPoint32TypeDef.ctl" = cluster{"Horizontal":i32, "Vertical":i32}
  T19 = typedef "OPC UA.lvlib/OPC Settings.ctl" = cluster{"Cycle Period":dbl, "server endpoint URL":string, "security policy":cluster{"message mode":enum16{"None", "Sign", "Sign and Encrypt"}, "security":enum16{"Basic256", "Basic128Rsa15"}}, "Trust Any Server":bool}
  T20 = typedef "OPC UA.lvlib/Variable Data Cluster.ctl" = cluster{"node ID":T2, "browse name":string, "status":T3, "timestamp":timestamp, "value ":variant}
  T21 = typedef "Subscription ID.ctl" = u32
  T22 = typedef "OPC UA Client Refnum.ctl" = refnum<k21>
  T23 = typedef "OPC UA.lvlib/OPC Tag Data.ctl" = cluster{"Include this Device":bool, "Device Name":string, "OPC Tag Data":cluster{"Tag":string, "Value":variant, "Time Stamp":timestamp}[]}
  T24 = typedef "Feed Module.lvlib/Feed Module Config Cluster.ctl" = cluster{"GUID":string, "Drop Coords":T18, "Process Name":string, "User name":string, "Queue Name":string, "Settings":T25, "Settings Load Count":i32, "OP Load Count":i32}
  T25 = typedef "Feed Module.lvlib/Feed Module Settings Cluster.ctl" = cluster{"Cycle Period":dbl, "Ismatech":T26, "Masterflex":T27, "Mettler":T28, "Bronkhorst M13 Flow Meter":T29, "PID 2 Parameters":T30, "Manual Entry":dbl, "Auto?":bool, "output range":cluster{"output high":dbl, "output low":dbl}, "Tacmina Settings":T33, "KNF SIMDOS Settings":T34, "ASIA Pump C":T35, "VICI Settings":T36, "FLOM Settings":T37, "SSI PR/LD Settings":T38, "Masterflex 75211 Settings":T39, "SSI P40 Settings":T40, "Ismatech 3 Channel Settings":T41, "Bronkhorst M14 Settings":T42}
  T26 = typedef "Ismatec ISM 831C.lvlib/Ismatech ISM831C Settings Cluster.ctl" = cluster{"VISA resource name":refnum<visa-resource-name>, "Simulated?":bool, "Pump Number":dbl, "Reverse?":bool}
  T27 = typedef "Masterflex 7550-30.lvlib/Settings Cluster.ctl" = cluster{"VISA resource name":refnum<visa-resource-name>, "Simulated?":bool, "Pump Number":dbl, "Reverse?":bool}
  T28 = typedef "Mettler Toledo.lvlib/Settings Cluster.ctl" = cluster{"VISA resource name":refnum<visa-resource-name>, "Simulated?":bool}
  T29 = typedef "Bronkhorst M13 Flow Meter.lvlib/Settings Cluster.ctl" = cluster{"VISA resource name":refnum<visa-resource-name>, "Simulated?":bool, "Smoothing Steps":i32}
  T30 = typedef "PID 2 Parameters Cluster.ctl" = cluster{"Input Device":T31, "Output Device":T32, "Setpoint":dbl, "PID gains":cluster{"proportional gain (Kc)":dbl, "integral time (Ti, min)":dbl, "derivative time (Td, min)":dbl}}
  T31 = typedef "PID Input Enum.ctl" = enum16{"Default", "Bronkhorst M13", "Bronkhorst M14", "Scale Rate of Change"}
  T32 = typedef "PID 2 Output Enum.ctl" = enum16{"Default", "Ismatec ISM 4308", "Ismatec ISM 831C", "Masterflex 7550-30", "VICI", "Tacmina QI", "KNF SIMDOS", "ASIA Type C", "FLOM UI-22-11", "SSI PR/LD", "SSI P40", "Masterflex 75211-70"}
  T33 = typedef "Tacmina QI.lvlib/Tacmina QI DAQ Setting.ctl" = cluster{"Analog DAQ Task":refnum<k21>, "Digital DAQ Task":refnum<k21>}
  T34 = typedef "KNF SIMDOS.lvlib/Settings Cluster plus SIMDOS.ctl" = cluster{"VISA resource name":refnum<visa-resource-name>, "Simulated?":bool}
  T35 = typedef "ASIA Pump.lvlib/Pump Settings.ctl" = cluster{"ASIA Pump #":i32, "channel":i32, "Simulated":bool}
  T36 = typedef "VICI M6 M50 Party Mode.lvlib/Settings Cluster.ctl" = cluster{"VISA resource name":refnum<visa-resource-name>, "Simulated?":bool, "Pump Letter":string, "Reverse?":bool}
  T37 = typedef "FLOM Pump.lvlib/Settings Cluster.ctl" = cluster{"VISA resource name":refnum<visa-resource-name>, "Simulated?":bool, "Pump Number":dbl}
  T38 = typedef "SSI PR or LD Pump.lvlib/SSI PR or LD Settings Cluster.ctl" = cluster{"VISA resource name":refnum<visa-resource-name>, "Simulated?":bool}
  T39 = typedef "Masterflex 75211.lvlib/Masterflex 75211 DAQ Setting.ctl" = cluster{"Analog DAQ Task":refnum<k21>, "Digital DAQ Task":refnum<k21>}
  T40 = typedef "SSI P40 Pump.lvlib/SSI P40 Settings Cluster.ctl" = cluster{"VISA resource name":refnum<visa-resource-name>, "Simulated?":bool}
  T41 = typedef "Ismatec 4308.lvlib/Ismatec 4083.ctl" = cluster{"VISA resource name":refnum<visa-resource-name>, "Pump Number":i16, "Channel Number":i16, "Simulated?":bool, "Reverse?":bool}
  T42 = typedef "Bronkhorst M14 Flow Meter.lvlib/Settings Cluster.ctl" = cluster{"VISA resource name":refnum<visa-resource-name>, "Simulated?":bool, "Smoothing Steps":i32}
  T43 = typedef "TT Module.lvlib/TT Module Config Cluster.ctl" = cluster{"GUID":string, "Drop Coords":T18, "Input Channel Tag Name ":string, "Process Name":string, "User name":string, "Queue Name":string, "Input Channel Numeric Alarm Settings":T44[]}
  T44 = typedef "Numeric Alarm Settings Cluster.ctl" = cluster{"enable? (F)":bool, "name":string, "alarm type":enum16{"HI_HI", "HI", "LO", "LO_LO"}, "level/change":dbl, "deadband/time":dbl, "alarm delay":dbl, "priority":u32, "ack type":enum16{"Auto", "User", "None", "Each Occurrence"}, "area":string, "description":string, "log? (T)":bool}
  T45 = typedef "DAQ.lvlib/Hardware Configuration.ctl" = cluster{"Tasks":T46[]}
  T46 = typedef "Task Cluster.ctl" = cluster{"DAQmx Task":refnum<k21>, "Read-Write Radio":enum32{"Read", "Write"}}
  T47 = typedef "PT Module.lvlib/PT Module Config Cluster.ctl" = cluster{"GUID":string, "Drop Coords":T18, "Input Channel Tag Name ":string, "Process Name":string, "User name":string, "Queue Name":string, "Input Channel Numeric Alarm Settings":T44[]}
  T48 = typedef "Scale Module.lvlib/Scale Module Config Cluster.ctl" = cluster{"GUID":string, "Drop Coords":T18, "Process Name":string, "User name":string, "Queue Name":string, "Settings":T49, "Load Count":i32}
  T49 = typedef "Scale Module.lvlib/Scale Module Settings Cluster.ctl" = cluster{"Cycle Period":dbl, "Mettler":T28, "Scale Type":string}
  T50 = typedef "Pump Module.lvlib/Pump Module Config Cluster.ctl" = cluster{"GUID":string, "Drop Coords":T18, "Process Name":string, "User name":string, "Queue Name":string, "Settings":T51, "Load Count":i32}
  T51 = typedef "Pump Module.lvlib/Pump Module Settings Cluster.ctl" = cluster{"Cycle Period":dbl, "Manual Entry":dbl, "Output Device":T32, "Ismatech":T26, "Ismatech 3 Channel Settings":T41, "Masterflex":T27, "VICI Settings":T36, "Tacmina Settings":T33, "KNF SIMDOS Settings":T34, "ASIA Pump C":T35, "FLOM Settings":T37, "SSI PR/LD Settings":T38, "SSI P40 Settings":T38, "Masterflex 75211 Settings":T39, "Pump Calibration File":path, "Calibration Slope":dbl, "Calibration Y Intercept":dbl, "Pump Cal Enum":u16}
  T52 = typedef "U3 Module.lvlib/U3 Module Config Cluster.ctl" = cluster{"GUID":string, "Drop Coords":T18, "AI Channel Number":enum16{"Default", "AI0", "AI1", "AI2", "AI3", "AI4", "AI5", "AI6", "AI7"}, "Process Name":string, "User name":string, "Queue Name":string, "Input Channel Numeric Alarm Settings":T44[]}
  T53 = typedef "Decoration Module Config Cluster.ctl" = cluster{"GUID":string, "Drop Coords":T18, "Decoration Filepath":path}
  T54 = typedef "Flow Module.lvlib/Flow Module Config Cluster.ctl" = cluster{"GUID":string, "Drop Coords":T18, "Process Name":string, "User name":string, "Queue Name":string, "Settings":T55, "Load Count":i32}
  T55 = typedef "Flow Module.lvlib/Flow Module Settings Cluster.ctl" = cluster{"Cycle Period":dbl, "Flow Meter Type":string, "Bronkhorst M13 Settings":T29, "Bronkhorst M14 Settings":T42}
  T56 = typedef "TCU Module.lvlib/TCU Module Config Cluster.ctl" = cluster{"GUID":string, "Drop Coords":T18, "Process Name":string, "User name":string, "Queue Name":string, "Settings":T57, "Load Count":i32, "Power Level Changed":bool}
  T57 = typedef "TCU Module.lvlib/TCU Module Settings Cluster.ctl" = cluster{"Cycle Period":dbl, "Setpoint Entry":dbl, "Output Device":T58, "Huber Ministat 230 Settings":T59, "Lauda Settings":T60, "Julabo FP-50 Settings":T61, "Internal Control?":bool, "Huber Unistat 410 Settings":T62}
  T58 = typedef "Output Devices.ctl" = enum16{"Default", "Huber Ministat 230", "Huber Unistat 410", "Lauda XT-150", "Julabo FP-50"}
  T59 = typedef "Huber Ministat 230 TCU.lvlib/Huber Settings.ctl" = cluster{"VISA resource name":refnum<visa-resource-name>, "Simulated?":bool}
  T60 = typedef "Lauda TCU.lvlib/Lauda Settings.ctl" = cluster{"VISA resource name":refnum<visa-resource-name>, "Simulated?":bool, "Pump Power":i32}
  T61 = typedef "Julabo Type FP-50 TCU.lvlib/Julabo FP-50 Settings.ctl" = cluster{"VISA resource name":refnum<visa-resource-name>, "Simulated?":bool, "Pump Power":i32}
  T62 = typedef "Huber Unistat 410 TCU.lvlib/Huber Unistat 410 RS485 Settings.ctl" = cluster{"VISA resource name":refnum<visa-resource-name>, "Address":i8, "Simulated?":bool}
  T63 = typedef "Not Sure Where this is Used.ctl" = T64[]
  T64 = typedef "Sequencing Library.lvlib/Squence Control.ctl" = cluster{"Module":string, "Control":u16, "Value":dbl, "Wait (sec)":dbl}
  T65 = typedef "D-O Module.lvlib/D-O Module Config Cluster.ctl" = cluster{"GUID":string, "Drop Coords":T18, "Process Name":string, "User name":string, "Queue Name":string, "Settings":T66, "Load Count":i32}
  T66 = typedef "D-O Module.lvlib/Valve Clusters.ctl" = cluster{"Valve Settings":T67, "Valve Type":enum16{"Default", "Digital Output Valve", "VICI Electronic Actuator"}, "Time On (Sec)":dbl, "Time Off (Sec)":dbl, "Run?":bool}
  T67 = typedef "D-O Module.lvlib/D-O Module Settings Cluster.ctl" = cluster{"D-O Settings":T68, "VICI Electronic Actuator":T69}
  T68 = typedef "D-O Module.lvlib/D-O Device Settings Cluster.ctl" = cluster{"DAQmx Task Name":refnum<k21>, "Output Channel":u16, "Output Channel Names":string[]}
  T69 = typedef "VICI Electronic Actuator.lvlib/VICI Electronic Actuator Settings.ctl" = cluster{"VISA resource name":refnum<visa-resource-name>, "Mode":enum16{"Two Positions With Stops", "Two Positions Without Stops", "Mutiposition"}, "Simulated":bool}
  T70 = typedef "4-20mA Module.lvlib/4-20mA Module Config Cluster.ctl" = cluster{"GUID":string, "Drop Coords":T18, "Process Name":string, "User name":string, "Queue Name":string, "Settings":T71, "Settings Load Count":i32}
  T71 = typedef "4-20mA Module.lvlib/4-20mA Module Settings Cluster.ctl" = cluster{"Cycle Period":dbl, "PID 2 Parameters":cluster{"Input Device":enum16{"Default", "4-20mA"}, "Output Device":enum16{"Default", "Equilibar Pressure Reg", "Flow Regulator"}, "Setpoint":dbl, "PID gains":cluster{"proportional gain (Kc)":dbl, "integral time (Ti, min)":dbl, "derivative time (Td, min)":dbl}, "output range":cluster{"output low":dbl, "output high":dbl}}, "Manual Entry":dbl, "Auto?":bool, "4-20mA Input Settings":T72, "4-20mA Out Settings":T73, "Input Channel Tag Name ":string}
  T72 = typedef "Pressure Transmitter Library.lvlib/Pressure Transmitter Device Settings.ctl" = cluster{"Input Channel ":u16}
  T73 = typedef "Pressure Regulator Library.lvlib/Pressure Regulator Device Settings.ctl" = cluster{"Output DAQ Task":refnum<k21>}
  T74 = typedef "Sonicator Module.lvlib/Sonicator Module Config Cluster.ctl" = cluster{"GUID":string, "Drop Coords":T18, "Process Name":string, "User name":string, "Queue Name":string, "Settings":T75, "Load Count":i32}
  T75 = typedef "Sonicator Module.lvlib/Sonicator Module Settings Cluster.ctl" = cluster{"Cycle Period":dbl, "Sonicator Type":string, "SS P100 Settings":T76, "Setpoint (µm)":dbl, "Cutoff (W)":dbl}
  T76 = typedef "Sonic Systems P100.lvlib/Sonic Systems P100 Settings.ctl" = cluster{"VISA resource name":refnum<visa-resource-name>, "Simulated?":bool}
  T77 = typedef "Agitator Module.lvlib/Agitator Module Config Cluster.ctl" = cluster{"GUID":string, "Drop Coords":T18, "Process Name":string, "User name":string, "Queue Name":string, "Settings":T78, "Load Count":i32}
  T78 = typedef "Agitator Module.lvlib/Agitator Module Settings Cluster.ctl" = cluster{"Cycle Period":dbl, "Agitator Type":string, "Setpoint (µm)":dbl}
  T79 = typedef "Main Queue Cluster.ctl" = cluster{"UI":refnum<queue>, "Waveform Loop":refnum<queue>, "CSV Log":refnum<queue>, "TDMS Log":refnum<queue>, "Graphs":refnum<queue>[], "DAQ":refnum<queue>, "Sequence":refnum<queue>, "TCP Write":refnum<queue>, "Sequence UI":refnum<queue>, "OPC UA Log":refnum<queue>, "TCP Read":refnum<queue>}
  T80 = typedef "Supported Security Policies.ctl" = cluster{"None":bool, "Sign with Basic128Rsa15":bool, "Sign and Encrypt with Basic128Rsa15":bool, "Sign with Basic256":bool, "Sign and Encrypt with Basic256":bool}
  T81 = typedef "OPC UA Variable Node Refnum.ctl" = refnum<k21>
  T82 = cluster{"property node ID":T2, "OPC UA variable node refnum out":T81, "name":string}[]
  T83 = typedef "OPC UA Server Refnum.ctl" = refnum<k21>
  T84 = typedef "Write Variant Request.ctl" = cluster{"node ID":T2, "value":variant, "timestamp (current time)":timestamp, "node status":T85}
  T85 = typedef "Write Status.ctl" = u32
  T86 = cluster{"node ID":T2, "value":i32, "timestamp (current time)":timestamp, "node status":T85}[]
  T87 = typedef "NodeIds.ctl" = T2[]
  T88 = cluster{"reference type":u32, "node ID":T2, "browse name":string, "node class":T4, "node type":u32}[]
  T89 = cluster{"property node ID":T2, "OPC UA variable node refnum out":T81, "name":string}
  T90 = cluster{"name":string, "data type":T8, "access level":u16, "description":string}
  T91 = typedef "Tag FGV Operation Enum.ctl" = enum16{"Init", "Set Notification Queue", "Create Tag", "Commit", "Write Tag (Numeric)", "Write Tag (Boolean)", "Read All Tags", "Read One Tag", "Delete Tag Category", "Set Alarm Parameters (Numeric)", "Set Alarm Parameters (Boolean)", "Enable All Alarms", "Disable All Alarms", "Delete All Tags", "Read Alarms", "Ack Alarm", "Read Alarm Parameters (Numeric)", "Read Alarm Parameters (Boolean)"}
  T92 = typedef "Module Tags Array Cluster.ctl" = cluster{"Feed Module Tags Array":T93[], "TT Tags Array":T94[], "PT Tags Array":T95[], "DAQ Tags Array":string[], "Scale Tags Array":cluster{"Scale Value":string, "Scale Error":string, "Identifier Tag":string}[], "Pump Module Tags Array":T96[], "Flow Module Tags Array":T97[], "TCU Module Tags Array":T98[], "DO Tags Array":T99[], "PR Module Tags Array":T100[], "OPC Module Tags Array":T101[], "Sonicator Module Tags Array":T102[], "AM Module Tags Array":T103[]}
  T93 = typedef "Feed Module.lvlib/Feed Module Tag Names Cluster.ctl" = cluster{"Pump Flow Tag":string, "PID 2 Out Tag":string, "Identifier Tag":string, "Scale Tag":string, "Density Tag":string, "FL Temp":string, "Input Device Tag":string, "Output Device Tag":string, "Pump's Flow":string, "Pump's Pressure":string, "Overpressure Tag":string}
  T94 = typedef "TT Module.lvlib/TT Module Tag Names.ctl" = cluster{"Temperature Value":string, "Identifier Tag":string}
  T95 = typedef "PT Module.lvlib/PT Module Tag Names.ctl" = cluster{"Pressure Value":string, "Identifier Tag":string}
  T96 = typedef "Pump Module.lvlib/Pump Module Tag Names Cluster.ctl" = cluster{"Pump Speed":string, "Pump Flow":string, "Pump Pressure":string, "Output Device Tag":string, "Overpressure Tag":string, "Identifier Tag":string}
  T97 = typedef "Flow Module.lvlib/Tag Cluster.ctl" = cluster{"Flow Tag":string, "Input Disconnected":string, "Density Tag":string, "Temp Tag":string, "Identifier Tag":string}
  T98 = typedef "TCU Module.lvlib/TCU Module Tag Names Cluster.ctl" = cluster{"TCU Temp":string, "Output Device Tag":string, "TCU Speed":string, "Identifier Tag":string}
  T99 = typedef "D-O Module.lvlib/D-O Module Tag Names Cluster.ctl" = cluster{"D-O Status":string, "Identifier Tag":string}
  T100 = typedef "4-20mA Module.lvlib/4-20mA Module Tag Names Cluster.ctl" = cluster{"4-20mA Input":string, "PID 2 Out Tag":string, "4-20mA Output":string, "Input Device Tag":string, "Output Device Tag":string, "Identifier Tag":string}
  T101 = typedef "OPC Module Tag Names.ctl" = cluster{"Output Device Tag":string, "Data Name Array":string[], "Identifier Tag":string}
  T102 = typedef "Sonicator Module.lvlib/Sonicator Module Tag Names.ctl" = cluster{"Amplitude Tag":string, "Power Tag":string, "Output Device Tag":string, "Identifier Tag":string}
  T103 = typedef "Agitator Module.lvlib/Agitator Module Tag Names.ctl" = cluster{"Amplitude Tag":string, "Power Tag":string, "Output Device Tag":string, "Identifier Tag":string}
  T104 = cluster{"Scale Value":string, "Scale Error":string, "Identifier Tag":string}[]
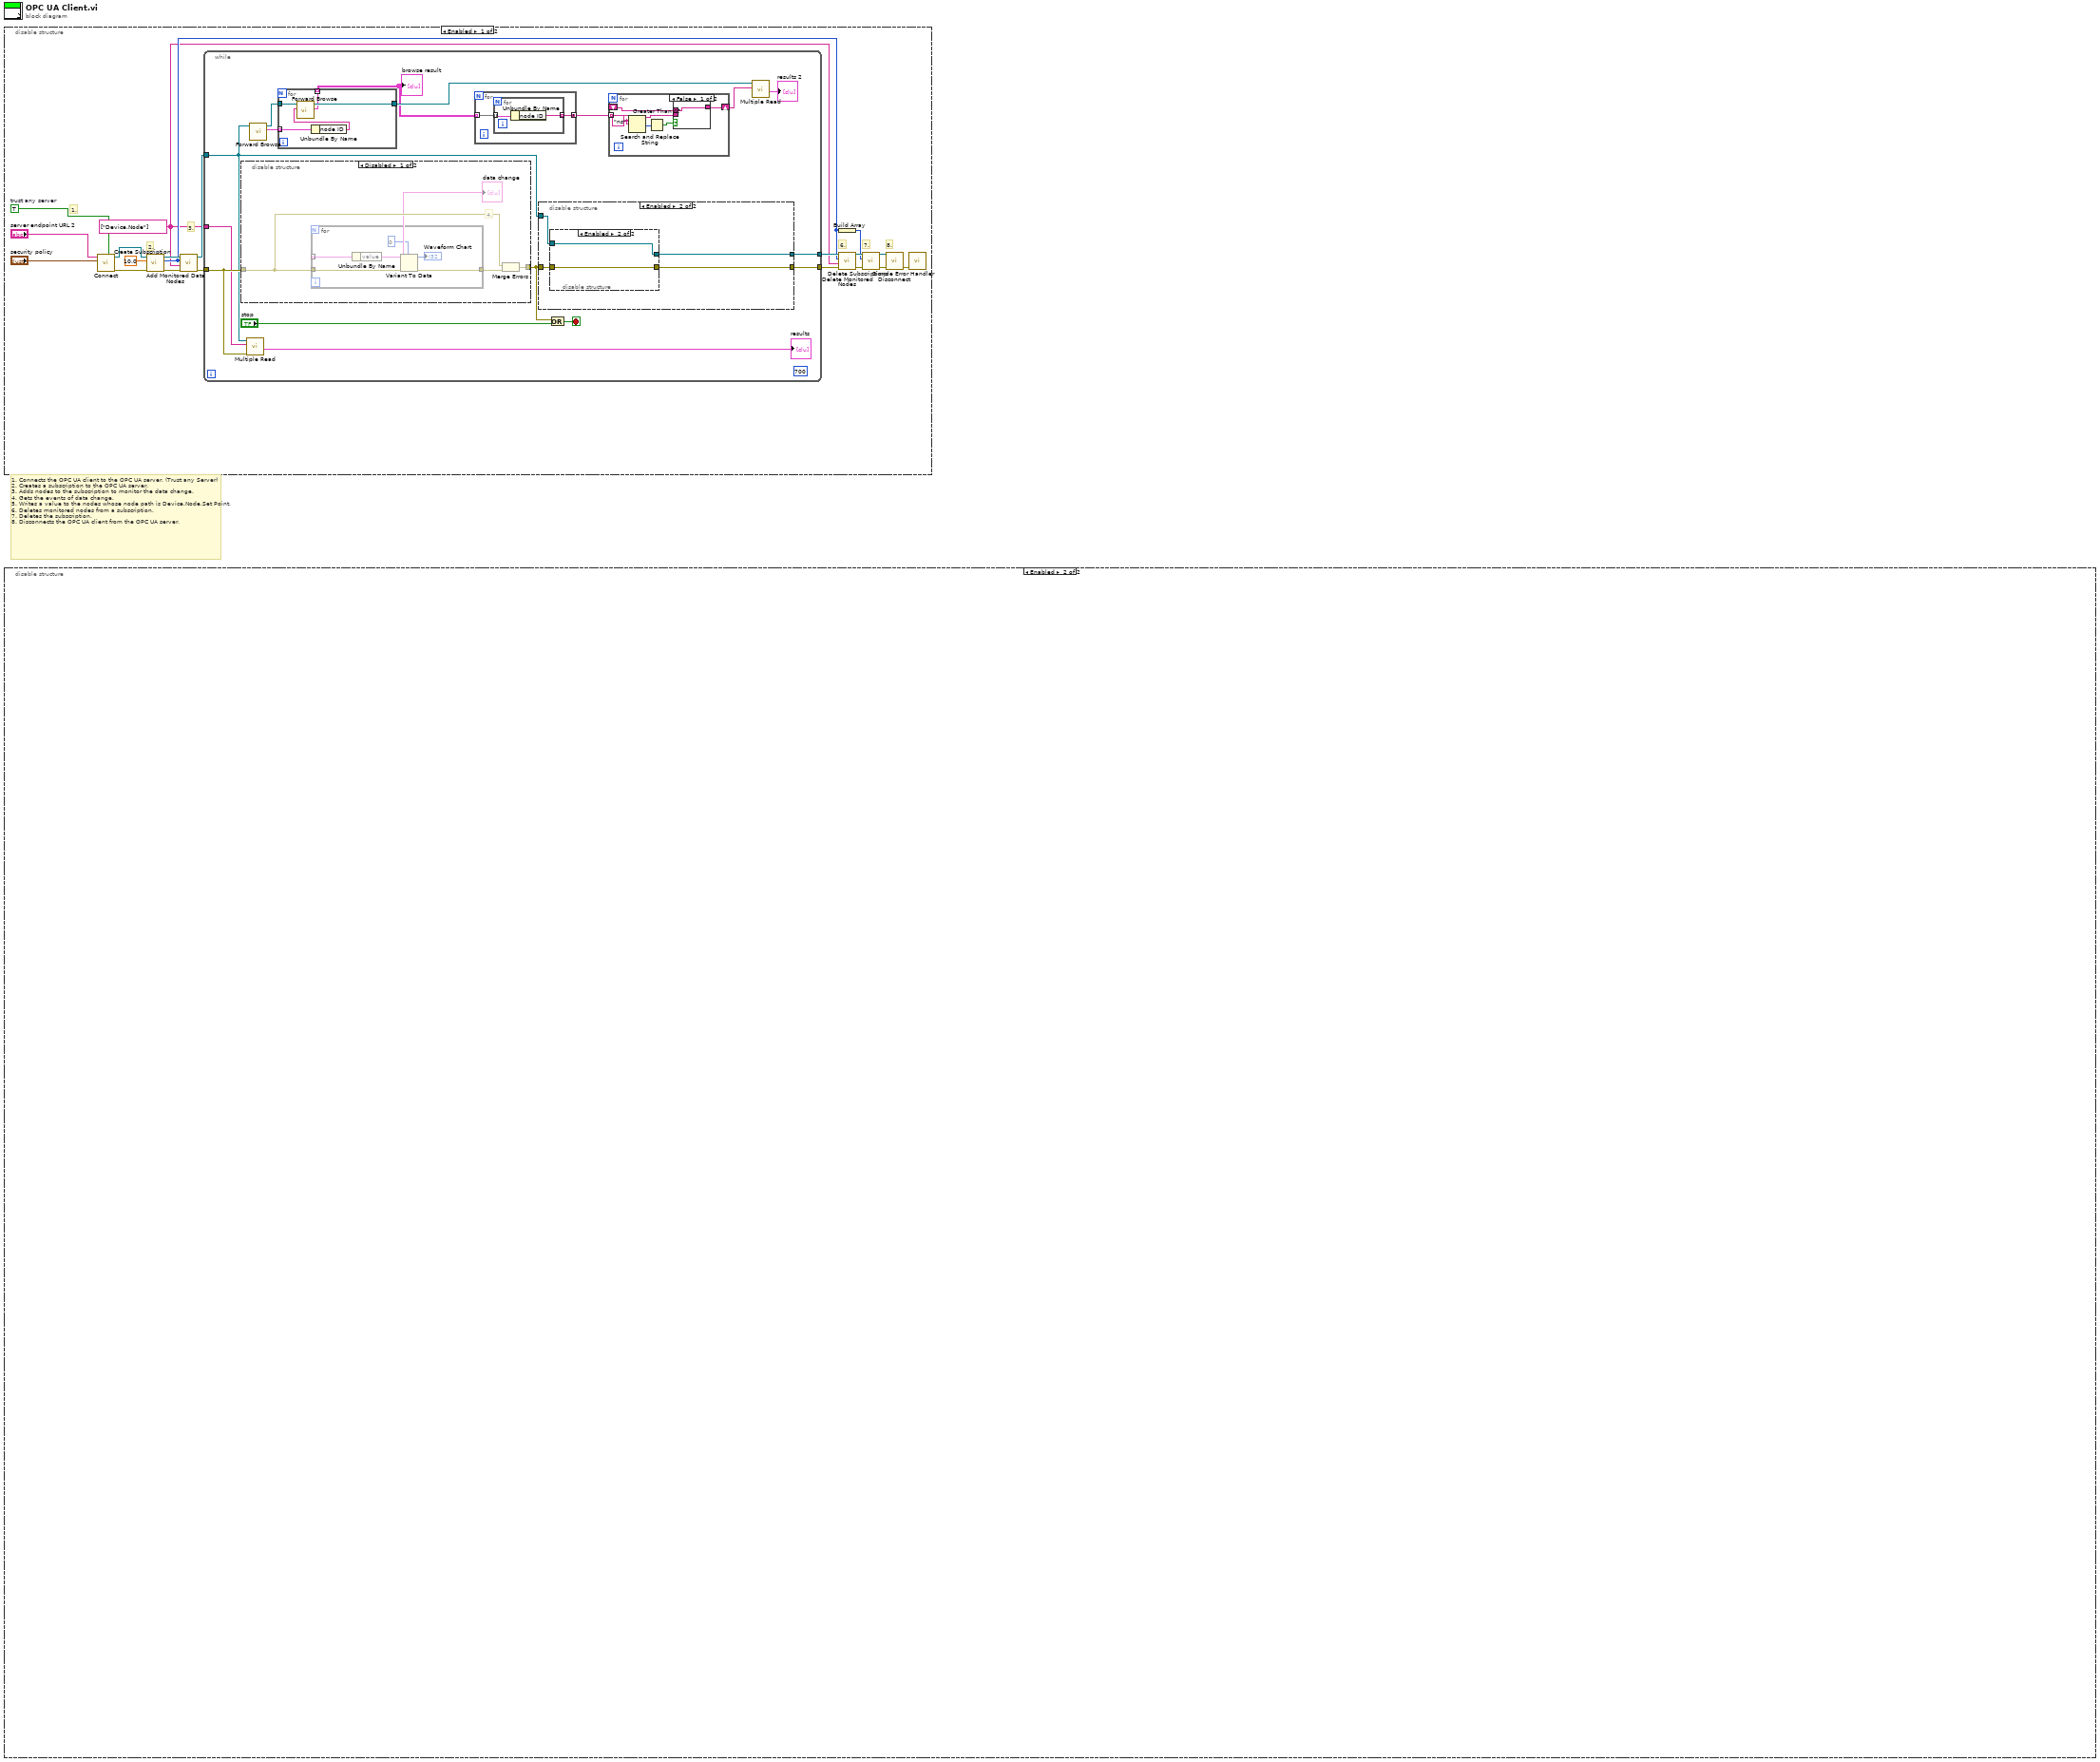
[diagram p0: block diagram]
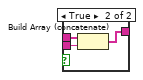
[diagram p2: hidden frame]
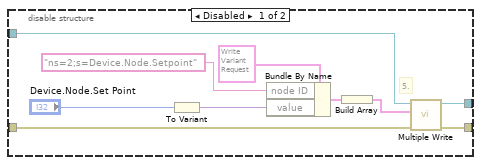
[diagram p4: hidden frame]
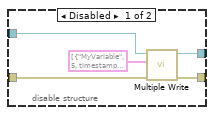
[diagram p5: hidden frame]
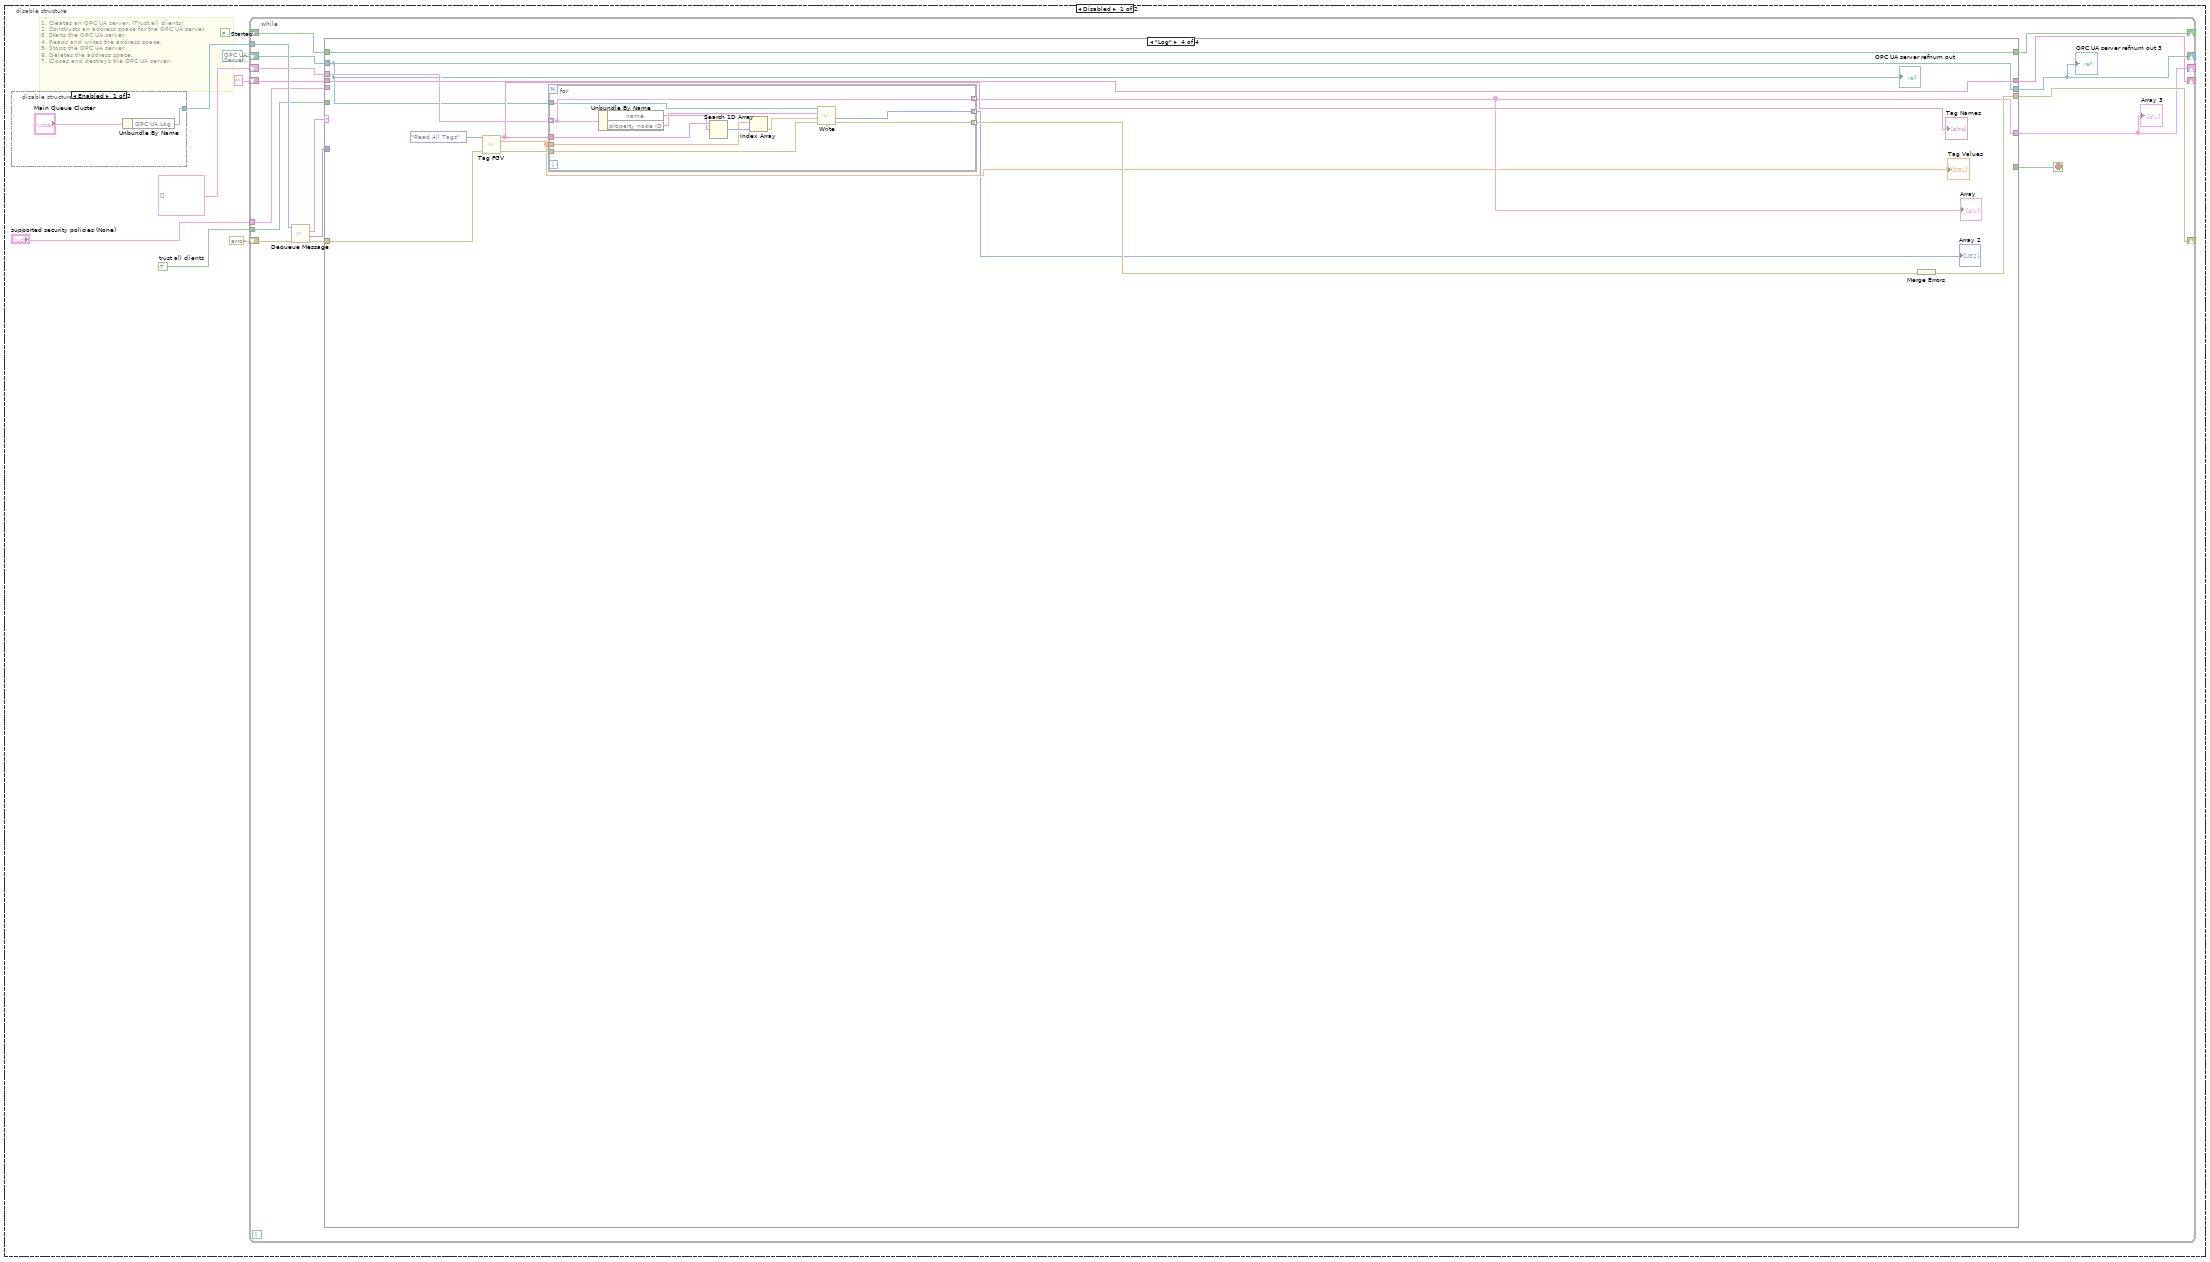
[diagram p7: hidden frame]
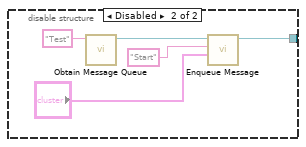
[diagram p8: hidden frame]
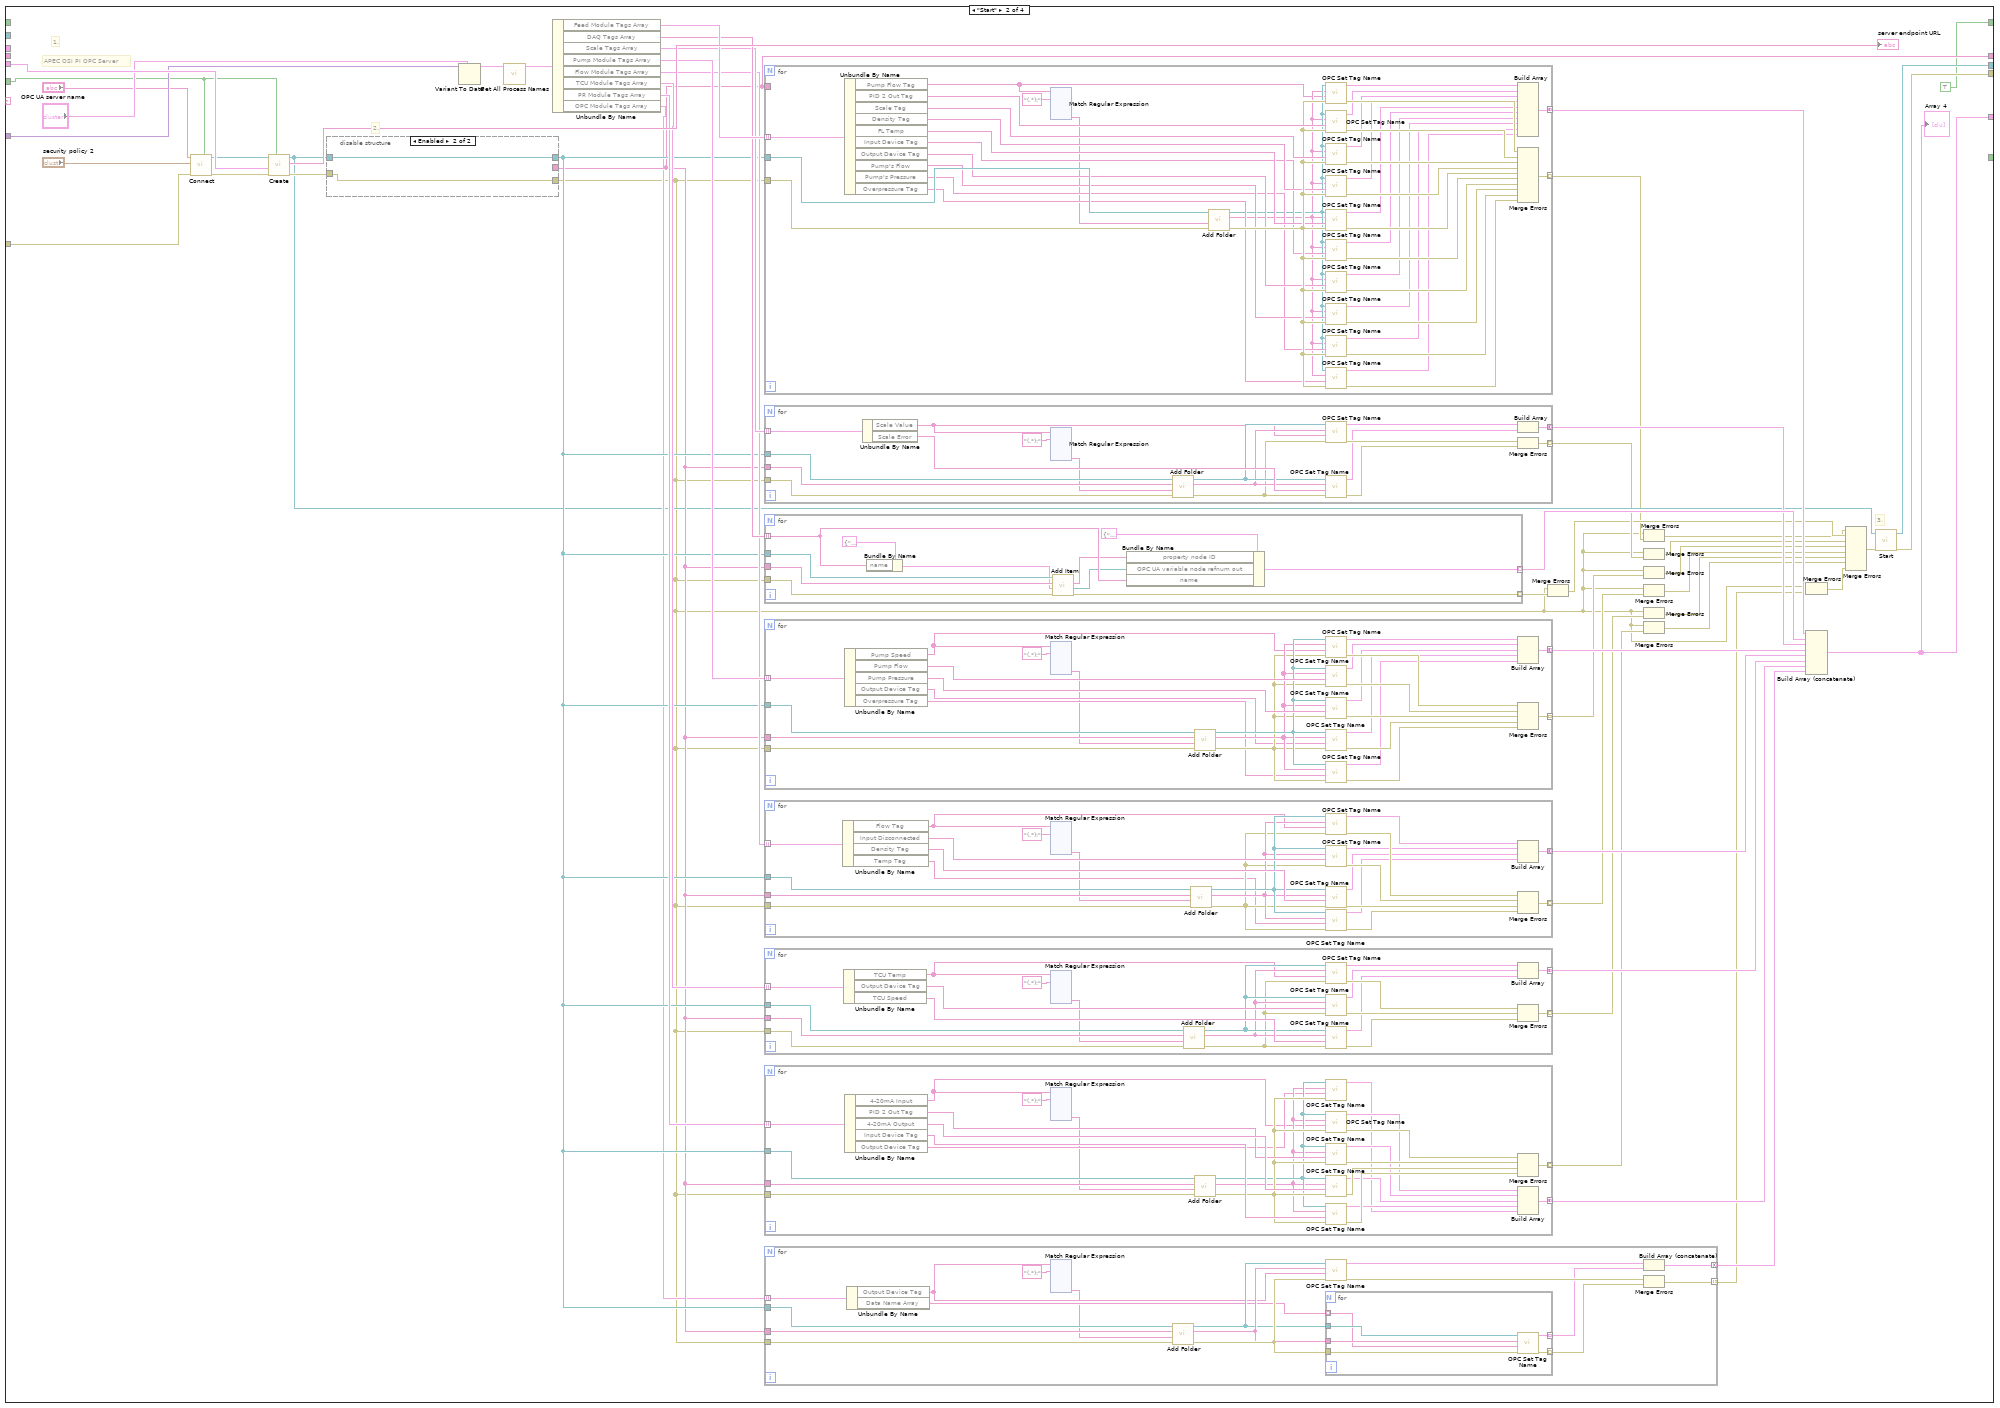
[diagram p10: hidden frame]
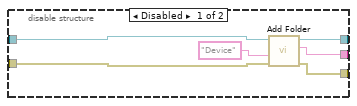
[diagram p11: hidden frame]
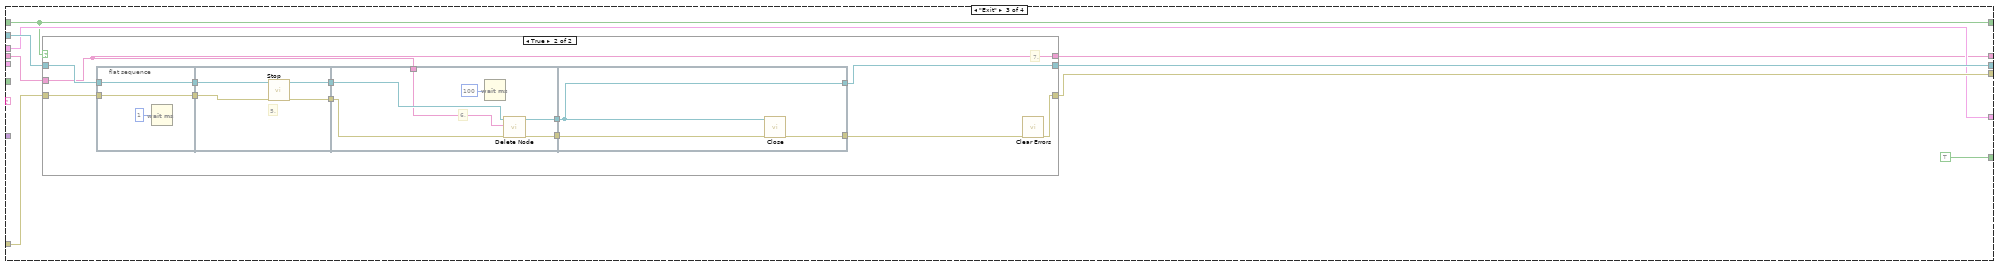
[diagram p12: hidden frame]
diagram:
  # "1. Connects the OPC UA client to the OPC UA server. (Trust any Server) \n2. Creates a subscription to the OPC UA server.\n3. Adds nodes to the subscription to monitor the data change.\n4. Gets the events of data change.\n5. Writes a value to the nodes whose node path is Device.Node.Set Point. \n6. Deletes monitored nodes from a subscription.\n7. Deletes the subscription.\n8. Disconnects the OPC UA client from the OPC UA server."
  n1 = disable-structure shown="Enabled" {
    frame Enabled {
      w2 = TRUE  # trust any server
      w1 = T87 ["Device.Node"] ("node IDs")
      # "7."
      # "8."
      # "6."
      # "3."
      # "2."
      # "1."
      n2 = call <vilib>:"Connect.vi"("trust any server (F)"=w2, "security policy"="security policy", "server endpoint URL"="server endpoint URL 2") -> ("error out"=w8:errorcluster, "OPC UA client refnum out"=w9:T22)  [unwired: 6 in, 1 out]
      n3 = call <vilib>:"Create Subscription.vi"("error in (no error)"=w8, "publishing interval (1000 ms)"=10.0 ("update rate (1000 ms)"), "OPC UA client refnum in"=w9) -> ("error out"=w18:errorcluster, "subscription ID out"=w6:T21, "OPC UA client refnum out"=w19:T22)  [unwired: 4 in, 2 out]
      n4 = call <vilib>:"Add Monitored Data Nodes.vi"("error in (no error)"=w18, "node IDs"=w1, "subscription ID in"=w6, "OPC UA client refnum in"=w19) -> ("error out"=w16:errorcluster, "OPC UA client refnum out"=w17:T22)  [unwired: 4 in, 2 out]
      n5 = while {
        tunnel: w17 -> [w28]
        tunnel: w16 -> [w31]
        tunnel: [w35] -> w14
        tunnel: [w36] -> w15
        tunnel: w1 -> [w29]
        stop <- w32 stop-if-true
        (unwired) 700
        n6 = disable-structure shown="Disabled" {
          disable-tunnel: [w60 w67] -> w34
          disable-tunnel: w31 -> [w58 w67]
          frame Disabled {
            # "4."
            n7 = for {
              tunnel: "data change" -> [w66] mode=indexing
              tunnel: w58 -> [w62]
              tunnel: [w61] -> w59
              n8 = Unbundle By Name(w66) -> ("value"=w65)
              n9 = Variant To Data(error in=w62, type=0, Variant=w65) -> (data=→"Waveform Chart":i32, error out=w61:errorcluster)
            }
            n10 = Merge Errors(w58, w59) -> (w60:errorcluster)
          }
          frame Enabled {
          }
        }
        n11 = call-poly <vilib>:"Multiple Read.vi"("error in (no error)"=w31, "node IDs"=w29, "OPC UA client refnum in"=w28) -> ("results"=→"results":T1[])  [unwired: 5 in, 3 out]
        n12 = call <vilib>:"Forward Browse.vi"("OPC UA client refnum in"=w28) -> ("browse result"=w27:T88, "OPC UA client refnum out"=w26:T22)  [unwired: 7 in, 2 out]
        n13 = for {
          tunnel: w27 -> [w56] mode=indexing
          tunnel: w26 -> [w55]
          tunnel: [w52] -> w23 mode=indexing
          tunnel: [w53] -> w25
          n14 = Unbundle By Name(w56) -> ("node ID"=w54:T2)
          n15 = call <vilib>:"Forward Browse.vi"("node ID"=w54, "OPC UA client refnum in"=w55) -> ("browse result"=w52:T88, "OPC UA client refnum out"=w53:T22)  [unwired: 6 in, 2 out]
        }
        "browse result" <- w23
        n16 = for {
          tunnel: w23 -> [w49] mode=indexing
          tunnel: [w48] -> w22 mode=concatenating
          n17 = for {
            tunnel: w49 -> [w51] mode=indexing
            tunnel: [w50] -> w48 mode=indexing
            n18 = Unbundle By Name(w51) -> ("node ID"=w50:T2)
          }
        }
        n19 = disable-structure shown="Enabled" {
          disable-tunnel: w28 -> [w77 w79]
          disable-tunnel: [w76 w81] -> w36
          disable-tunnel: [w75 w80] -> w35
          disable-tunnel: w34 -> [w68 w78]
          frame Disabled {
            # "5."
            n20 = To Variant(anything="Device.Node.Set Point") -> (Variant=w73:variant)
            n21 = Bundle By Name(cluster=T84 {"node ID"="", "value"=variant, "timestamp (current time)"=timestamp(0 s since 1904-01-01), "node status"=0} ("request"), "node ID"=T2 "ns=2;s=Device.Node.Setpoint", "value"=w73) -> (w70:T84)
            n22 = Build Array(w70) -> (w69:T84[])
            n23 = call-poly <vilib>:"Multiple Write.vi"("error in (no error)"=w68, "requests"=w69, "OPC UA client refnum in"=w77) -> ("error out"=w75:errorcluster, "OPC UA client refnum out"=w76:T22)  [unwired: 5 in, 2 out]
          }
          frame Enabled {
            n24 = disable-structure shown="Enabled" {
              disable-tunnel: [w86 w87] -> w81
              disable-tunnel: [w85 w88] -> w80
              disable-tunnel: w79 -> [w84 w87]
              disable-tunnel: w78 -> [w83 w88]
              frame Disabled {
                n25 = call-poly <vilib>:"Multiple Write.vi"("error in (no error)"=w83, "requests"=T86 [{"node ID"="MyVariable", "value"=5, "timestamp (current time)"=timestamp(0 s since 1904-01-01), "node status"=0}], "OPC UA client refnum in"=w84) -> ("error out"=w85:errorcluster, "OPC UA client refnum out"=w86:T22)  [unwired: 5 in, 2 out]
              }
              frame Enabled {
              }
            }
          }
        }
        n26 = Compound Arithmetic op=OR(w34, "stop") -> (w32:bool)
        n27 = for {
          tunnel: w22 -> [w41] mode=indexing
          shift-right: [w39] -> w21
          shift-left: _ -> [w40]
          w43 = "ns" ("search string")
          n28 = Search and Replace String(input string=w41, search string=w43, replace string=w43) -> (result string=w38:string, number of replacements=w42:i32)  [unwired: 5 in, 2 out]
          n29 = Greater Than 0?(x=w42) -> (x > 0?=w37:bool)
          n30 = case shown="False" w37 {
            tunnel: w40 -> [w44 w47]
            tunnel: [w44 w46] -> w39
            tunnel: w38 -> [_ w45]
            frame False {
            }
            frame True {
              n31 = Build Array (concatenate)(w47, w45) -> (w46:string[])
            }
          }
        }
        n32 = call-poly <vilib>:"Multiple Read.vi"("node IDs"=w21, "OPC UA client refnum in"=w25) -> ("results"=→"results 2":T1[])  [unwired: 6 in, 3 out]
      }
      n33 = Build Array(w6) -> (w5:T21[])
      n34 = call <vilib>:"Delete Monitored Nodes.vi"("error in (no error)"=w14, "node IDs"=w1, "subscription ID in"=w6, "OPC UA client refnum in"=w15) -> ("error out"=w12:errorcluster, "OPC UA client refnum out"=w13:T22)  [unwired: 3 in, 3 out]
      n35 = call <vilib>:"Delete Subscriptions.vi"("error in (no error)"=w12, "subscription IDs"=w5, "OPC UA client refnum in"=w13) -> ("error out"=w10:errorcluster, "OPC UA client refnum out"=w11:T22)  [unwired: 6 in, 1 out]
      n36 = call <vilib>:"Disconnect.vi"("error in (no error)"=w10, "OPC UA client refnum in"=w11) -> ("error out"=w3:errorcluster)  [unwired: 9 in]
      n37 = call <vilib>:"Simple Error Handler.vi"("error in (no error)"=w3) -> ()  [unwired: 4 in, 5 out]
    }
    frame Disabled {
    }
  }
  n38 = disable-structure shown="Enabled" {
    frame Disabled {
      w89 = FALSE  # Started
      w96 = TRUE  # trust all clients
      # "1. Creates an OPC UA server. (Trust all clients)\n2. Constructs an address space for the OPC UA server.\n3. Starts the OPC UA server.\n4. Reads and writes the address space.\n5. Stops the OPC UA server.\n6. Deletes the address space.\n7. Closes and destroys the OPC UA server."
      n39 = disable-structure shown="Enabled" {
        disable-tunnel: [w98 w100] -> w94
        frame Enabled {
          n40 = Unbundle By Name("Main Queue Cluster") -> ("OPC UA Log"=w98:refnum<queue>)
        }
        frame Disabled {
          n41 = call "Obtain Message Queue.vi"("name (unnamed)"="Test") -> ("Message Queue"=w99:refnum<queue>)  [unwired: 9 in, 1 out]
          n42 = call-poly "Enqueue Message.vi"("Message Data"="?", "Message"="Start", "Message Queue"=w99) -> ("dup Message Queue"=w100:refnum<queue>)  [unwired: 7 in, 1 out]
        }
      }
      n43 = while {
        tunnel: w94 -> [w119]
        shift-right: [w116] -> _
        shift-left: errorcluster {"status"=FALSE, "code"=0, "source"=""} ("error IO") -> [w115]
        tunnel: w96 -> [w114]
        tunnel: "supported security policies (None)" -> [w113]
        shift-right: [w112] -> _
        shift-left: T83 refnum ("OPC UA server refnum out") -> [w111]
        shift-right: [w110] -> _
        shift-left: T2 "" ("folder node ID") -> [w108]
        shift-right: [w107] -> _
        shift-left: T82 [] -> [w106]
        shift-right: [w105] -> _
        shift-left: w89 -> [w104]
        stop <- w118 stop-if-true
        n44 = call "Dequeue Message.vi"("error in (no error)"=w115, "Message Queue"=w119) -> ("error out"=w117:errorcluster, "Message Data"=w109:variant, "Message"=w120:string)  [unwired: 6 in, 1 out]
        n45 = case shown="\"Log\"" w120 {
          tunnel: [_ _ TRUE _] -> w118
          tunnel: w117 -> [w123 w129 w1185 w1234]
          tunnel: [w123 w176 w1192 w1229] -> w116
          tunnel: w114 -> [_ w130 _ _]
          tunnel: w113 -> [_ w178 _ _]
          tunnel: [w124 w177 w1190 w1225] -> w112
          tunnel: w111 -> [w124 _ w1191 w1225]
          tunnel: [w125 w153 w1186 w1235] -> w110
          tunnel: w109 -> [_ w174 _ _]
          tunnel: w108 -> [w125 _ w1189 w1235]
          tunnel: [w122 w132 w1188 w1231] -> w107
          tunnel: w106 -> [w122 _ w1188 w1232]
          tunnel: w104 -> [w121 _ w1187 w1226]
          tunnel: [w121 TRUE ("Started") w1187 w1226] -> w105
          frame Default {
          }
          frame "Start" {
            # "APEC OSI PI OPC Server"
            # "3."
            # "2."
            # "1."
            n46 = call <vilib>:"Connect.vi"("trust any server (F)"=w130, "error in (no error)"=w129, "security policy"="security policy 2", "server endpoint URL"="OPC UA server name") -> ("error out"=w126:errorcluster, "OPC UA client refnum out"=w127:T22)  [unwired: 5 in, 1 out]
            n47 = call <vilib>:"Create.vi"("trust all clients (F)"=w130, "error in (no error)"=w126, "supported security policies (None)"=w178, "OPC UA server name"=w127) -> ("error out"=w175:errorcluster, "server endpoint URL"=→"server endpoint URL":string, "OPC UA server refnum out"=w151:T83)  [unwired: 5 in]
            n48 = disable-structure shown="Enabled" {
              disable-tunnel: w175 -> [w185 w186]
              disable-tunnel: [w183 w187] -> w154
              disable-tunnel: [w182 _] -> w153
              disable-tunnel: [w181 w186] -> w134
              disable-tunnel: w151 -> [w180 w187]
              frame Disabled {
                n49 = call <vilib>:"Add Folder.vi"("error in (no error)"=w185, "folder name"="Device", "OPC UA server refnum in"=w180) -> ("error out"=w181:errorcluster, "folder node ID"=w182:T2, "OPC UA server refnum out"=w183:T83)  [unwired: 5 in]
              }
              frame Enabled {
              }
            }
            n50 = Variant To Data(type="?", Variant=w174) -> (data=w172:T9)  [unwired: 1 in, 1 out]
            n51 = call "Get All Process Names.vi"(11:w172) -> ("Module Tags Array Cluster"=w170:T92)  [unwired: 9 in, 1 out]
            n52 = Unbundle By Name(w170) -> ("Feed Module Tags Array"=w171:T93[], "DAQ Tags Array"=w169:string[], "Scale Tags Array"=w167:T104, "Pump Module Tags Array"=w166:T96[], "Flow Module Tags Array"=w165:T97[], "TCU Module Tags Array"=w164:T98[], "PR Module Tags Array"=w163:T100[], "OPC Module Tags Array"=w152:T101[])
            n53 = for {
              tunnel: w134 -> [w1068]
              tunnel: w153 -> [_]
              tunnel: w154 -> [w1067]
              tunnel: [w1065] -> w135 mode=indexing
              tunnel: w171 -> [w1066] mode=indexing
              tunnel: [w1034] -> w162 mode=concatenating
              n54 = Unbundle By Name(w1066) -> ("Pump Flow Tag"=w1030:string, "PID 2 Out Tag"=w1063:string, "Scale Tag"=w1064:string, "Density Tag"=w1058:string, "FL Temp"=w1057:string, "Input Device Tag"=w1056:string, "Output Device Tag"=w1055:string, "Pump's Flow"=w1054:string, "Pump's Pressure"=w1053:string, "Overpressure Tag"=w1052:string)
              n55 = xnode "Match Regular Expression"("input string"=w1030, "regular expression"="(.*):") -> ("submatch 1"=w1029:string)  [unwired: 4 in, 5 out]
              n56 = call <vilib>:"Add Folder.vi"("error in (no error)"=w1068, "folder name"=w1029, "OPC UA server refnum in"=w1067) -> ("error out"=w1059:errorcluster, "folder node ID"=w1032:T2, "OPC UA server refnum out"=w1033:T83)  [unwired: 5 in]
              n57 = call "OPC Set Tag Name.vi"("error in (no error)"=w1059, "name"=w1030, "item node ID"=w1032, "Refnum in"=w1033) -> ("error out"=w1062:errorcluster, "OPC Property cluster"=w1044:T89)  [unwired: 6 in]
              n58 = call "OPC Set Tag Name.vi"("error in (no error)"=w1059, "name"=w1063, "item node ID"=w1032, "Refnum in"=w1033) -> ("error out"=w1061:errorcluster, "OPC Property cluster"=w1043:T89)  [unwired: 6 in]
              n59 = call "OPC Set Tag Name.vi"("error in (no error)"=w1059, "name"=w1064, "item node ID"=w1032, "Refnum in"=w1033) -> ("error out"=w1060:errorcluster, "OPC Property cluster"=w1042:T89)  [unwired: 6 in]
              n60 = call "OPC Set Tag Name.vi"("error in (no error)"=w1059, "name"=w1058, "item node ID"=w1032, "Refnum in"=w1033) -> ("error out"=w1051:errorcluster, "OPC Property cluster"=w1041:T89)  [unwired: 6 in]
              n61 = call "OPC Set Tag Name.vi"("error in (no error)"=w1059, "name"=w1057, "item node ID"=w1032, "Refnum in"=w1033) -> ("error out"=w1050:errorcluster, "OPC Property cluster"=w1040:T89)  [unwired: 6 in]
              n62 = call "OPC Set Tag Name.vi"("error in (no error)"=w1059, "name"=w1056, "item node ID"=w1032, "Refnum in"=w1033) -> ("error out"=w1049:errorcluster, "OPC Property cluster"=w1039:T89)  [unwired: 6 in]
              n63 = call "OPC Set Tag Name.vi"("error in (no error)"=w1059, "name"=w1055, "item node ID"=w1032, "Refnum in"=w1033) -> ("error out"=w1048:errorcluster, "OPC Property cluster"=w1038:T89)  [unwired: 6 in]
              n64 = call "OPC Set Tag Name.vi"("error in (no error)"=w1059, "name"=w1054, "item node ID"=w1032, "Refnum in"=w1033) -> ("error out"=w1047:errorcluster, "OPC Property cluster"=w1037:T89)  [unwired: 6 in]
              n65 = call "OPC Set Tag Name.vi"("error in (no error)"=w1059, "name"=w1053, "item node ID"=w1032, "Refnum in"=w1033) -> ("error out"=w1046:errorcluster, "OPC Property cluster"=w1036:T89)  [unwired: 6 in]
              n66 = call "OPC Set Tag Name.vi"("error in (no error)"=w1059, "name"=w1052, "item node ID"=w1032, "Refnum in"=w1033) -> ("error out"=w1045:errorcluster, "OPC Property cluster"=w1035:T89)  [unwired: 6 in]
              n67 = Build Array(w1044, w1043, w1042, w1041, w1040, w1039, w1038, w1037, w1036, w1035) -> (w1034:T82)
              n68 = Merge Errors(w1062, w1061, w1060, w1051, w1050, w1049, w1048, w1047, w1046, w1045) -> (w1065:errorcluster)
            }
            n69 = for {
              tunnel: [w900] -> w139 mode=indexing
              tunnel: w167 -> [w901] mode=indexing
              tunnel: w154 -> [w893]
              tunnel: w153 -> [w892]
              tunnel: w134 -> [w891]
              tunnel: [w888] -> w160 mode=concatenating
              n70 = Unbundle By Name(w901) -> ("Scale Value"=w886:string, "Scale Error"=w899:string)
              n71 = xnode "Match Regular Expression"("input string"=w886, "regular expression"="(.*):") -> ("submatch 1"=w885:string)  [unwired: 4 in, 5 out]
              n72 = call <vilib>:"Add Folder.vi"("error in (no error)"=w891, "folder name"=w885, "parent folder node ID"=w892, "OPC UA server refnum in"=w893) -> ("error out"=w894:errorcluster, "folder node ID"=w895:T2, "OPC UA server refnum out"=w896:T83)  [unwired: 4 in]
              n73 = call "OPC Set Tag Name.vi"("error in (no error)"=w894, "name"=w886, "item node ID"=w895, "Refnum in"=w896) -> ("error out"=w898:errorcluster, "OPC Property cluster"=w890:T89)  [unwired: 6 in]
              n74 = call "OPC Set Tag Name.vi"("error in (no error)"=w894, "name"=w899, "item node ID"=w895, "Refnum in"=w896) -> ("error out"=w897:errorcluster, "OPC Property cluster"=w889:T89)  [unwired: 6 in]
              n75 = Build Array(w890, w889) -> (w888:T82)
              n76 = Merge Errors(w898, w897) -> (w900:errorcluster)
            }
            n77 = for {
              tunnel: w134 -> [w1028]
              tunnel: w153 -> [w1027]
              tunnel: w154 -> [w1026]
              tunnel: [w1023] -> w137 mode=indexing
              tunnel: w169 -> [w1021] mode=indexing
              tunnel: [w1018] -> w161 mode=indexing
              n78 = Bundle By Name(cluster=T90 {"name"="Node", "data type"=11, "access level"=3, "description"=""} ("item"), "name"=w1021) -> (w1024:T90)
              n79 = call <vilib>:"Add Item.vi"("error in (no error)"=w1028, "item"=w1024, "parent folder node ID"=w1027, "OPC UA server refnum in"=w1026) -> ("error out"=w1023:errorcluster, "OPC UA variable node refnum out"=w1020:T81, "item node ID"=w1019:T2)  [unwired: 3 in, 1 out]
              n80 = Bundle By Name(cluster=T89 {"property node ID"="", "OPC UA variable node refnum out"="", "name"=""} ("OPC Property cluster"), "property node ID"=w1019, "OPC UA variable node refnum out"=w1020, "name"=w1021) -> (w1018:T89)
            }
            n81 = for {
              tunnel: w134 -> [w768]
              tunnel: w153 -> [w767]
              tunnel: w154 -> [w766]
              tunnel: [w746] -> w141 mode=indexing
              tunnel: w166 -> [w765] mode=indexing
              tunnel: [w747] -> w159 mode=concatenating
              n82 = Unbundle By Name(w765) -> ("Pump Speed"=w744:string, "Pump Flow"=w763:string, "Pump Pressure"=w764:string, "Output Device Tag"=w756:string, "Overpressure Tag"=w755:string)
              n83 = xnode "Match Regular Expression"("input string"=w744, "regular expression"="(.*):") -> ("submatch 1"=w743:string)  [unwired: 4 in, 5 out]
              n84 = call <vilib>:"Add Folder.vi"("error in (no error)"=w768, "folder name"=w743, "parent folder node ID"=w767, "OPC UA server refnum in"=w766) -> ("error out"=w757:errorcluster, "folder node ID"=w758:T2, "OPC UA server refnum out"=w759:T83)  [unwired: 4 in]
              n85 = call "OPC Set Tag Name.vi"("error in (no error)"=w757, "name"=w744, "item node ID"=w758, "Refnum in"=w759) -> ("error out"=w762:errorcluster, "OPC Property cluster"=w752:T89)  [unwired: 6 in]
              n86 = call "OPC Set Tag Name.vi"("error in (no error)"=w757, "name"=w763, "item node ID"=w758, "Refnum in"=w759) -> ("error out"=w761:errorcluster, "OPC Property cluster"=w751:T89)  [unwired: 6 in]
              n87 = call "OPC Set Tag Name.vi"("error in (no error)"=w757, "name"=w764, "item node ID"=w758, "Refnum in"=w759) -> ("error out"=w760:errorcluster, "OPC Property cluster"=w750:T89)  [unwired: 6 in]
              n88 = call "OPC Set Tag Name.vi"("error in (no error)"=w757, "name"=w756, "item node ID"=w758, "Refnum in"=w759) -> ("error out"=w754:errorcluster, "OPC Property cluster"=w749:T89)  [unwired: 6 in]
              n89 = call "OPC Set Tag Name.vi"("error in (no error)"=w757, "name"=w755, "item node ID"=w758, "Refnum in"=w759) -> ("error out"=w753:errorcluster, "OPC Property cluster"=w748:T89)  [unwired: 6 in]
              n90 = Build Array(w752, w751, w750, w749, w748) -> (w747:T82)
              n91 = Merge Errors(w762, w761, w760, w754, w753) -> (w746:errorcluster)
            }
            n92 = for {
              tunnel: w134 -> [w626]
              tunnel: w153 -> [w625]
              tunnel: w154 -> [w624]
              tunnel: [w622] -> w143 mode=indexing
              tunnel: w165 -> [w623] mode=indexing
              tunnel: [w607] -> w158 mode=concatenating
              n93 = Unbundle By Name(w623) -> ("Flow Tag"=w605:string, "Input Disconnected"=w620:string, "Density Tag"=w621:string, "Temp Tag"=w613:string)
              n94 = xnode "Match Regular Expression"("input string"=w605, "regular expression"="(.*):") -> ("submatch 1"=w604:string)  [unwired: 4 in, 5 out]
              n95 = call <vilib>:"Add Folder.vi"("error in (no error)"=w626, "folder name"=w604, "parent folder node ID"=w625, "OPC UA server refnum in"=w624) -> ("error out"=w614:errorcluster, "folder node ID"=w615:T2, "OPC UA server refnum out"=w616:T83)  [unwired: 4 in]
              n96 = call "OPC Set Tag Name.vi"("error in (no error)"=w614, "name"=w605, "item node ID"=w615, "Refnum in"=w616) -> ("error out"=w619:errorcluster, "OPC Property cluster"=w611:T89)  [unwired: 6 in]
              n97 = call "OPC Set Tag Name.vi"("error in (no error)"=w614, "name"=w620, "item node ID"=w615, "Refnum in"=w616) -> ("error out"=w618:errorcluster, "OPC Property cluster"=w610:T89)  [unwired: 6 in]
              n98 = call "OPC Set Tag Name.vi"("error in (no error)"=w614, "name"=w621, "item node ID"=w615, "Refnum in"=w616) -> ("error out"=w617:errorcluster, "OPC Property cluster"=w609:T89)  [unwired: 6 in]
              n99 = call "OPC Set Tag Name.vi"("error in (no error)"=w614, "name"=w613, "item node ID"=w615, "Refnum in"=w616) -> ("error out"=w612:errorcluster, "OPC Property cluster"=w608:T89)  [unwired: 6 in]
              n100 = Build Array(w611, w610, w609, w608) -> (w607:T82)
              n101 = Merge Errors(w619, w618, w617, w612) -> (w622:errorcluster)
            }
            n102 = for {
              tunnel: w134 -> [w487]
              tunnel: w153 -> [w486]
              tunnel: w154 -> [w485]
              tunnel: [w483] -> w145 mode=indexing
              tunnel: w164 -> [w484] mode=indexing
              tunnel: [w471] -> w157 mode=concatenating
              n103 = Unbundle By Name(w484) -> ("TCU Temp"=w468:string, "Output Device Tag"=w481:string, "TCU Speed"=w482:string)
              n104 = xnode "Match Regular Expression"("input string"=w468, "regular expression"="(.*):") -> ("submatch 1"=w469:string)  [unwired: 4 in, 5 out]
              n105 = call <vilib>:"Add Folder.vi"("error in (no error)"=w487, "folder name"=w469, "parent folder node ID"=w486, "OPC UA server refnum in"=w485) -> ("error out"=w475:errorcluster, "folder node ID"=w476:T2, "OPC UA server refnum out"=w477:T83)  [unwired: 4 in]
              n106 = call "OPC Set Tag Name.vi"("error in (no error)"=w475, "name"=w468, "item node ID"=w476, "Refnum in"=w477) -> ("error out"=w480:errorcluster, "OPC Property cluster"=w474:T89)  [unwired: 6 in]
              n107 = call "OPC Set Tag Name.vi"("error in (no error)"=w475, "name"=w481, "item node ID"=w476, "Refnum in"=w477) -> ("error out"=w479:errorcluster, "OPC Property cluster"=w473:T89)  [unwired: 6 in]
              n108 = call "OPC Set Tag Name.vi"("error in (no error)"=w475, "name"=w482, "item node ID"=w476, "Refnum in"=w477) -> ("error out"=w478:errorcluster, "OPC Property cluster"=w472:T89)  [unwired: 6 in]
              n109 = Build Array(w474, w473, w472) -> (w471:T82)
              n110 = Merge Errors(w480, w479, w478) -> (w483:errorcluster)
            }
            n111 = for {
              tunnel: w134 -> [w351]
              tunnel: w153 -> [w350]
              tunnel: w154 -> [w349]
              tunnel: [w347] -> w147 mode=indexing
              tunnel: w163 -> [w348] mode=indexing
              tunnel: [w330] -> w156 mode=concatenating
              n112 = Unbundle By Name(w348) -> ("4-20mA Input"=w328:string, "PID 2 Out Tag"=w345:string, "4-20mA Output"=w346:string, "Input Device Tag"=w340:string, "Output Device Tag"=w336:string)
              n113 = xnode "Match Regular Expression"("input string"=w328, "regular expression"="(.*):") -> ("submatch 1"=w327:string)  [unwired: 4 in, 5 out]
              n114 = call <vilib>:"Add Folder.vi"("error in (no error)"=w351, "folder name"=w327, "parent folder node ID"=w350, "OPC UA server refnum in"=w349) -> ("error out"=w339:errorcluster, "folder node ID"=w337:T2, "OPC UA server refnum out"=w338:T83)  [unwired: 4 in]
              n115 = call "OPC Set Tag Name.vi"("error in (no error)"=w339, "name"=w336, "item node ID"=w337, "Refnum in"=w338) -> ("OPC Property cluster"=w331:T89)  [unwired: 6 in, 1 out]
              n116 = call "OPC Set Tag Name.vi"("error in (no error)"=w339, "name"=w328, "item node ID"=w337, "Refnum in"=w338) -> ("error out"=w344:errorcluster, "OPC Property cluster"=w335:T89)  [unwired: 6 in]
              n117 = call "OPC Set Tag Name.vi"("error in (no error)"=w339, "name"=w345, "item node ID"=w337, "Refnum in"=w338) -> ("error out"=w343:errorcluster, "OPC Property cluster"=w334:T89)  [unwired: 6 in]
              n118 = call "OPC Set Tag Name.vi"("error in (no error)"=w339, "name"=w346, "item node ID"=w337, "Refnum in"=w338) -> ("error out"=w342:errorcluster, "OPC Property cluster"=w333:T89)  [unwired: 6 in]
              n119 = call "OPC Set Tag Name.vi"("error in (no error)"=w339, "name"=w340, "item node ID"=w337, "Refnum in"=w338) -> ("error out"=w341:errorcluster, "OPC Property cluster"=w332:T89)  [unwired: 6 in]
              n120 = Merge Errors(w344, w343, w342, w341) -> (w347:errorcluster)
              n121 = Build Array(w335, w334, w333, w332, w331) -> (w330:T82)
            }
            n122 = for {
              tunnel: w134 -> [w204]
              tunnel: w153 -> [w203]
              tunnel: w154 -> [w202]
              tunnel: [w200] -> w149 mode=indexing
              tunnel: w152 -> [w201] mode=indexing
              tunnel: [w197] -> w155 mode=concatenating
              n123 = Unbundle By Name(w201) -> ("Output Device Tag"=w189:string, "Data Name Array"=w192:string[])
              n124 = xnode "Match Regular Expression"("input string"=w189, "regular expression"="(.*):") -> ("submatch 1"=w188:string)  [unwired: 4 in, 5 out]
              n125 = call <vilib>:"Add Folder.vi"("error in (no error)"=w204, "folder name"=w188, "parent folder node ID"=w203, "OPC UA server refnum in"=w202) -> ("error out"=w196:errorcluster, "folder node ID"=w195:T2, "OPC UA server refnum out"=w194:T83)  [unwired: 4 in]
              n126 = call "OPC Set Tag Name.vi"("error in (no error)"=w196, "name"=w189, "item node ID"=w195, "Refnum in"=w194) -> ("error out"=w199:errorcluster, "OPC Property cluster"=w198:T89)  [unwired: 6 in]
              n127 = for {
                tunnel: w196 -> [w326]
                tunnel: w195 -> [w325]
                tunnel: w194 -> [w324]
                tunnel: [w323] -> w193 mode=indexing
                tunnel: w192 -> [w322] mode=indexing
                tunnel: [w321] -> w191 mode=indexing
                n128 = call "OPC Set Tag Name.vi"("error in (no error)"=w326, "name"=w322, "item node ID"=w325, "Refnum in"=w324) -> ("error out"=w323:errorcluster, "OPC Property cluster"=w321:T89)  [unwired: 6 in]
              }
              n129 = Build Array (concatenate)(w198, w191) -> (w197:T82)
              n130 = Merge Errors(w199, w193) -> (w200:errorcluster)
            }
            n131 = Merge Errors(w134, w137) -> (w136:errorcluster)
            n132 = Merge Errors(w134, w135) -> (w133:errorcluster)
            n133 = Merge Errors(w134, w139) -> (w138:errorcluster)
            n134 = Merge Errors(w134, w141) -> (w140:errorcluster)
            n135 = Merge Errors(w134, w143) -> (w142:errorcluster)
            n136 = Merge Errors(w134, w145) -> (w144:errorcluster)
            n137 = Merge Errors(w134, w147) -> (w146:errorcluster)
            n138 = Merge Errors(w134, w149) -> (w148:errorcluster)
            n139 = Build Array (concatenate)(w162, w161, w160, w159, w158, w157, w156, w155) -> (w132:T82)
            "Array 4" <- w132
            n140 = Merge Errors(w133, w136, w138, w140, w142, w144, w146, w148) -> (w168:errorcluster)
            n141 = call <vilib>:"Start.vi"("error in (no error)"=w168, "OPC UA server refnum in"=w151) -> ("error out"=w176:errorcluster, "OPC UA server refnum out"=w177:T83)  [unwired: 7 in, 1 out]
          }
          frame "Exit" {
            n142 = case shown="True" w1187 {
              tunnel: w1185 -> [w1195 w1208]
              tunnel: [w1195 w1197] -> w1192
              tunnel: w1191 -> [w1196 w1207]
              tunnel: [w1196 w1203] -> w1190
              tunnel: w1189 -> [w1194 w1204]
              tunnel: [w1194 w1204] -> w1186
              frame False {
              }
              frame True {
                # "7."
                n143 = flat-sequence {
                  tunnel: w1207 -> [w1210]
                  tunnel: w1208 -> [w1211]
                  tunnel: [w1211] -> w1200
                  tunnel: [w1210] -> w1199
                  tunnel: [w1215] -> w1206
                  tunnel: [w1214] -> w1205
                  tunnel: w1200 -> [w1213]
                  tunnel: w1199 -> [w1212]
                  tunnel: w1206 -> [w1221]
                  tunnel: w1205 -> [w1220]
                  tunnel: w1204 -> [w1219]
                  tunnel: [w1218] -> w1202
                  tunnel: [w1217] -> w1201
                  tunnel: [w1224] -> w1203
                  tunnel: w1202 -> [w1223]
                  tunnel: w1201 -> [w1224]
                  tunnel: [w1222] -> w1198
                  frame #0 {
                    n144 = Wait (ms)(milliseconds to wait=u32 1) -> ()  [unwired: 1 out]
                  }
                  frame #1 {
                    # "5."
                    n145 = call <vilib>:"Stop.vi"("error in (no error)"=w1213, "OPC UA server refnum in"=w1212) -> ("error out"=w1214:errorcluster, "OPC UA server refnum out"=w1215:T83)  [unwired: 8 in]
                  }
                  frame #2 {
                    # "6."
                    n146 = Wait (ms)(milliseconds to wait=u32 100) -> ()  [unwired: 1 out]
                    n147 = call <vilib>:"Delete Node.vi"("error in (no error)"=w1220, "node ID"=w1219, "OPC UA server refnum in"=w1221) -> ("error out"=w1218:errorcluster, "OPC UA server refnum out"=w1217:T83)  [unwired: 7 in]
                  }
                  frame #3 {
                    n148 = call <vilib>:"Close.vi"("error in (no error)"=w1223, "OPC UA server refnum in"=w1224) -> ("error out"=w1222:errorcluster)  [unwired: 9 in]
                  }
                }
                n149 = call <vilib>:"Clear Errors.vi"("error in (no error)"=w1198) -> ("error out"=w1197:errorcluster)  [unwired: 5 in, 1 out]
              }
            }
          }
          frame "Log" {
            n150 = call "Tag FGV.vi"("Operation"=Tag_FGV_Operation_Enum."Read All Tags", "error in (no error)"=w1234) -> ("Tag Names"=w1236:string[], "Tag Values"=w1228:dbl[], "error out"=w1233:errorcluster)  [unwired: 6 in, 5 out]
            "Tag Values" <- w1228
            "Tag Names" <- w1236
            n151 = for {
              tunnel: w1236 -> [w1247]
              tunnel: w1233 -> [w1242]
              tunnel: w1232 -> [w1248] mode=indexing
              tunnel: [w1248] -> w1231 mode=indexing
              tunnel: w1225 -> [w1243]
              tunnel: [w1241] -> w1230 mode=indexing
              tunnel: w1228 -> [w1240]
              tunnel: [w1238] -> w1227 mode=indexing
              n152 = Unbundle By Name(w1248) -> ("name"=w1246:string, "property node ID"=w1244:T2)
              n153 = Search 1D Array(1D array=w1247, element=w1246) -> (index of element=w1245:i32)  [unwired: 1 in]
              n154 = Index Array(array=w1240, index=w1245) -> (element=w1239:dbl)
              n155 = call-poly <vilib>:"Write.vi"("error in (no error)"=w1242, "value"=w1239, "node ID"=w1244, "OPC UA server refnum in"=w1243) -> ("error out"=w1241:errorcluster, "status"=w1238:T3)  [unwired: 5 in, 1 out]
            }
            "Array" <- w1231
            "Array 2" <- w1227
            n156 = Merge Errors(w1230) -> (w1229:errorcluster)
            "OPC UA server refnum out" <- w1225
          }
        }
        "OPC UA server refnum out 3" <- w112
        "Array 3" <- w107
      }
    }
    frame Enabled {
    }
  }
